vi "NOSAMSBouncerDAQ.vi"() -> (2 "Summary Data":T7 {"C12LE" format="%_3e"; "C13LE" format="%_3e"; "C1312" format="%_3e"; "C12" format="%_3e"; "C13L" format="%_3e"; "C13H" format="%_3e"}, 3 "Run Average Ratios":T8 {"LEC13/12" format="%_4e"; "DTfrac" format="%#_3g"; "DT" format="%#_3g"; "CountErr" format="%#_3g"; "d13C" format="%_4g"; "C13/12" format="%_4e"; "C14/12" format="%_4e"; "C14/13" format="%_3e"; "C12Cor" format="%_3e"; "C13" format="%_3e"; "C13H/L" format="%#_3g"})   [LabVIEW 2013]
uses:
  ctl/RunRatios.ctl
  ctl/SummaryData.ctl
  ctl/RunParameters.ctl
  ctl/PixieKeithleyDAQstates.ctl
  ctl/FCOffset.ctl
  ctl/BouncerParameters.ctl
  <vilib>/Utility/miscctls.llb/LVRowAndColumnTypeDef.ctl
  <vilib>/Utility/error.llb/DialogType.ctl
  <vilib>/DAQmx/write.llb/DAQmx Write (Analog Wfm 1Chan NSamp).vi
  <vilib>/DAQmx/read.llb/DAQmx Read (Analog 1D Wfm NChan NSamp).vi
  <vilib>/DAQmx/read.llb/DAQmx Read (Counter U32 1Chan 1Samp).vi
  <vilib>/DAQmx/create/channels.llb/DAQmx Create Channel (CI-Count Edges).vi
  <vilib>/DAQmx/create/channels.llb/DAQmx Create Channel (AI-Voltage-Basic).vi
  <vilib>/DAQmx/configure/trigger.llb/DAQmx Start Trigger (Digital Edge).vi
  <vilib>/DAQmx/configure/timing.llb/DAQmx Timing (Sample Clock).vi
  <vilib>/DAQmx/create/channels.llb/DAQmx Create Channel (AO-Voltage-Basic).vi
  <vilib>/DAQmx/configure/timing.llb/DAQmx Timing (Use Waveform).vi
  <vilib>/DAQmx/create/channels.llb/DAQmx Create Channel (CO-Pulse Generation-Time).vi
  <vilib>/DAQmx/configure/timing.llb/DAQmx Timing (Implicit).vi
  <vilib>/DAQmx/miscellaneous.llb/DAQmx Fill In Error Info.vi
  lib/PixieDriver/PixieDriver.lvlib
  <resource>/objmgr/daqmx.rc
panel:
  in  "Clear":bool
  in  "AI Samples":i32=1000
  in  "AI rate":dbl=100000.0 format="%0.2f"
  in  "Run Parameters":T1={"Block time (s)"=0.1, "Max Runtime (s)"=10.0, "Max Counts"=100000, "C12 Limit"=-1.0, "Max BadBlocks"=0, "Tuning"=FALSE, "WarmupTime"=0.0, "Warmup"=FALSE} {"Block time (s)" min=0.0 max=100.0 step=0.1}
  out "wheelfile array":string[][](array[string])=[["0", "Alfa Aesar", "N/A", "B", "30000", "180", "10", "10", "1", "", "", "", "", "", "", "", ""], ["1", "OX-I", "GS-18039", "S", "30000", "180", "10", "11", "1", "", "", "", "", "", "", "", ""], ["2", "IAEA C-1", "HY-25820", "B", "30000", "180", "10", "10", "1", "", "", "", "", "", "", "", ""], ["3", "Mullin 20150838702", "WS-32919", "U", "30000", "180", "10", "10", "1", "", "", "", "", "", "", "", ""], ["4", "Mullin 20150838703", "WS-32920", "U", "30000", "180", "10", "10", "1", "", "", "", "", "", "", "", ""], ["5", "Mullin 20150868701", "WS-32921", "U", "30000", "180", "10", "10", "1", "", "", "", "", "", "", "", ""], ["6", "Weidman Mollusc C", "HY-25773", "SS", "30000", "180", "10", "10", "1", "", "", "", "", "", "", "", ""], ["7", "OX-I", "GS-18039", "S", "30000", "180", "10", "10", "1", "", "", "", "", "", "", "", ""], ["8", "Mullin 20150928701", "WS-32922", "U", "30000", "180", "10", "10", "1", "", "", "", "", "", "", "", ""], ["9", "Mullin 20150928702", "WS-32923", "U", "30000", "180", "10", "10", "1", "", "", "", "", "", "", "", ""], ["10", "Mullin 20150928703", "WS-32924", "U", "30000", "180", "10", "10", "1", "", "", "", "", "", "", "", ""], ["11", "OX-I solid", "OC-43664", "SS", "30000", "180", "10", "10", "1", "", "", "", "", "", "", "", ""], ["12", "Mullin 20150938701", "WS-32925", "U", "30000", "180", "10", "10", "1", "", "", "", "", "", "", "", ""], ["13", "Mullin 20150938702", "WS-32926", "U", "30000", "180", "10", "10", "1", "", "", "", "", "", "", "", ""], ["14", "OX-I", "GS-18039", "S", "30000", "180", "10", "10", "1", "", "", "", "", "", "", "", ""], ["15", "Mullin 20150938703", "WS-32927", "U", "30000", "180", "10", "10", "1", "", "", "", "", "", "", "", ""], ["16", "Mullin 20150938704", "WS-32928", "U", "30000", "180", "10", "10", "1", "", "", "", "", "", "", "", ""], ["17", "Jenkins 40403", "GS-18101", "U", "30000", "180", "10", "10", "1", "", "", "", "", "", "", "", ""], ["18", "TIRI K carbonate", "HY-25794", "SS", "30000", "180", "10", "10", "1", "", "", "", "", "", "", "", ""], ["19", "Jenkins 40402", "GS-18102", "U", "30000", "180", "10", "10", "1", "", "", "", "", "", "", "", ""], ["20", "Jenkins 50412", "GS-18103", "U", "30000", "180", "10", "10", "1", "", "", "", "", "", "", "", ""], ["21", "OX-I", "GS-18039", "S", "30000", "180", "10", "10", "1", "", "", "", "", "", "", "", ""], ["22", "Jenkins 50212", "GS-18104", "U", "30000", "180", "10", "10", "1", "", "", "", "", "", "", "", ""], ["23", "Jenkins 50211", "GS-18105", "U", "30000", "180", "10", "10", "1", "", "", "", "", "", "", "", ""], ["24", "Jenkins 50210", "GS-18106", "U", "30000", "180", "10", "10", "1", "", "", "", "", "", "", "", ""], ["25", "Jenkins 50209", "GS-18108", "U", "30000", "180", "10", "10", "1", "", "", "", "", "", "", "", ""], ["26", "Jenkins 50208", "GS-18109", "U", "30000", "180", "10", "10", "1", "", "", "", "", "", "", "", ""], ["27", "OX-I", "GS-18130", "S", "30000", "180", "10", "10", "1", "", "", "", "", "", "", "", ""], ["28", "Jenkins 50207", "GS-18110", "U", "30000", "180", "10", "10", "1", "", "", "", "", "", "", "", ""], ["29", "Jenkins 50206", "GS-18111", "U", "30000", "180", "10", "10", "1", "", "", "", "", "", "", "", ""], ["30", "Jenkins 50205", "GS-18112", "U", "30000", "180", "10", "10", "1", "", "", "", "", "", "", "", ""], ["31", "TIRI I travertine", "HY-25808", "SS", "30000", "180", "10", "10", "1", "", "", "", "", "", "", "", ""], ["32", "Jenkins 50204", "GS-18120", "U", "30000", "180", "10", "10", "1", "", "", "", "", "", "", "", ""], ["33", "OX-I", "GS-17825", "S", "30000", "180", "10", "10", "1", "", "", "", "", "", "", "", ""], ["34", "Jenkins 50203", "GS-18121", "U", "30000", "180", "10", "10", "1", "", "", "", "", "", "", "", ""], ["35", "Jenkins 50202", "GS-18122", "U", "30000", "180", "10", "10", "1", "", "", "", "", "", "", "", ""], ["36", "Jenkins 50612", "GS-18123", "U", "30000", "180", "10", "10", "1", "", "", "", "", "", "", "", ""], ["37", "TIRI K carbonate", "HY-25634", "SS", "30000", "180", "10", "10", "1", "", "", "", "", "", "", "", ""], ["38", "Jenkins 50201", "GS-18124", "U", "30000", "180", "10", "10", "1", "", "", "", "", "", "", "", ""], ["39", "IAEA C-1", "HY-25820", "B", "30000", "180", "10", "10", "1", "", "", "", "", "", "", "", ""]]
  in  "Autoscale":bool=TRUE
  out "Warmup":bool
  out "C13":dbl format="%_3g"
  out "Meas":i32[](array[numeric])
  out "Runlist":i32[][](array[numeric])=[[10, 11, 10, 10, 10, 10, 10, 10, 10, 10, 10, 10, 10, 10, 10, 10, 10, 10, 10, 10, 10, 10, 10, 10, 10, 10, 10, 10, 10, 10, 10, 10, 10, 10, 10, 10, 10, 10, 10, 10]]
  in  "Clear Charts":bool
  out "LE Currents":cluster{"C13LE":dbl, "C12LE":dbl}(graph)={"C13LE"=-117.27091239941238, "C12LE"=-99.48155029506408}
  out "Currents & Counts":cluster{"C14Rate":dbl, "C12":dbl, dbl}(graph)={"C14Rate"=308.7222261479474, "C12"=134.96605939238734, 127.32704646662468}
  out "Ratios":T2(graph)={"C14/12"=1.082744261664239e-12, "C14/12"=1.1652819041526944e-12, "d13C"=-56.910193732367055, "d13C"=-56.70877952735165}
  in  "C12LE 2":dbl=1000000.0
  in  "C13LE 2":dbl=100000000.0
  in  "C13 2":dbl=100000000.0
  in  "C12 2":dbl=1000000.0
  out "Pos":i32
  in  "RowAndCollumn":T3
  in  "Numeric":i32
  in  "Start Run":bool
  in  "Tab Control":T4(tab)=enum."Status"
  in  "Load wheel":bool
  in  "Run Order":i32[](listbox)
  in  "Source Auto-shutdown":bool=TRUE
  in  "Local Results Directory":path=path "C:/Users/ams254/Documents/Results"
  out "Results path":path=path "C:/Users/ams254/Documents/Results/USAMS050815R.txt"
  out "wheelname":string caption="Wheel name"
  in  "Server Results Directory":path=path "H:/USAMS/Results"
  in  "First Run\nWarmup Multiplier":dbl=1.0 format="%#_13g"
  out "Bouncer I":waveform(dbl)(graph)={"t0"=timestamp(3552044335.624893 s since 1904-01-01), "dt"=9.999999999999972e-06, "Y"=[], "attributes"=variant("NI_ChannelName"=variant(string "PXI1Slot4/ai4"), "NI_UnitDescription"=variant(string "Volts"))}
  in  "Settings File":path
  in  "LoadSettings":bool
  in  "SaveSettings":bool
  out "HE 12C Cup":waveform(dbl)(graph)={"t0"=timestamp(3552044335.624885 s since 1904-01-01), "dt"=9.999999999999972e-06, "Y"=[], "attributes"=variant("NI_ChannelName"=variant(string "PXI1Slot4/ai0"), "NI_UnitDescription"=variant(string "Volts"))}
  out "LE 12C Cup":waveform(dbl)(graph)={"t0"=timestamp(3552044335.6252913 s since 1904-01-01), "dt"=9.999999999999972e-06, "Y"=[], "attributes"=variant("NI_ChannelName"=variant(string "PXI1Slot4/ai3"), "NI_UnitDescription"=variant(string "Volts"))}
  out "LE 13C Cup":waveform(dbl)(graph)={"t0"=timestamp(3552044335.625891 s since 1904-01-01), "dt"=9.999999999999972e-06, "Y"=[], "attributes"=variant("NI_ChannelName"=variant(string "PXI1Slot4/ai3"), "NI_UnitDescription"=variant(string "Volts"))}
  out "Bouncer V":waveform(dbl)(graph)={"t0"=timestamp(3552044335.624893 s since 1904-01-01), "dt"=9.999999999999972e-06, "Y"=[], "attributes"=variant("NI_ChannelName"=variant(string "PXI1Slot4/ai4"), "NI_UnitDescription"=variant(string "Volts"))}
  in  "FC Offset":T5={"HE 12C Offset"=-1.3999999999999993e-07, "HE 13CL Offset"=-1.6999999999999996e-10, "HE 13CH Offset"=-1.0000000000000004e-10, "LE FC Scale"=11, "HE C12 Scale"=11, "HE C13 Scale"=18} {"HE C13 Scale" items=["500 mA/V", "200 mA/V", "100 mA/V", "50 mA/V", "20 mA/V", "10 mA/V", "5 mA/V", "2 mA/V", "1 mA/V", "500 uA/V", "200 uA/V", "100 uA/V", "50 uA/V", "20 uA/V", "10 uA/V", "5 uA/V", "2 uA/V", "1 uA/V", "500 nA/V", "200 nA/V", "100 nA/V", "50 nA/V", "20 nA/V", "10 nA/V", "5 nA/V", "2 nA/V", "1 nA/V", "500 pA/V", "200 pA/V", "100 pA/V", "50 pA/V", "20 pA/V", "10 pA/V", "5 pA/V", "2 pA/V", "1 pA/V", ""]; "HE C12 Scale" items=["500 mA/V", "200 mA/V", "100 mA/V", "50 mA/V", "20 mA/V", "10 mA/V", "5 mA/V", "2 mA/V", "1 mA/V", "500 uA/V", "200 uA/V", "100 uA/V", "50 uA/V", "20 uA/V", "10 uA/V", "5 uA/V", "2 uA/V", "1 uA/V", "500 nA/V", "200 nA/V", "100 nA/V", "50 nA/V", "20 nA/V", "10 nA/V", "5 nA/V", "2 nA/V", "1 nA/V", "500 pA/V", "200 pA/V", "100 pA/V", "50 pA/V", "20 pA/V", "10 pA/V", "5 pA/V", "2 pA/V", "1 pA/V", ""]; "LE FC Scale" items=["500 mA/V", "200 mA/V", "100 mA/V", "50 mA/V", "20 mA/V", "10 mA/V", "5 mA/V", "2 mA/V", "1 mA/V", "500 uA/V", "200 uA/V", "100 uA/V", "50 uA/V", "20 uA/V", "10 uA/V", "5 uA/V", "2 uA/V", "1 uA/V", "500 nA/V", "200 nA/V", "100 nA/V", "50 nA/V", "20 nA/V", "10 nA/V", "5 nA/V", "2 nA/V", "1 nA/V", "500 pA/V", "200 pA/V", "100 pA/V", "50 pA/V", "20 pA/V", "10 pA/V", "5 pA/V", "2 pA/V", "1 pA/V", ""]; "HE 13CH Offset" format="%.1e"; "HE 13CL Offset" format="%_2e"; "HE 12C Offset" format="%_2e"}
  out "HE 13 SUM":waveform(dbl)(graph)={"t0"=timestamp(3552044335.625587 s since 1904-01-01), "dt"=9.999999999999972e-06, "Y"=[], "attributes"=variant("NI_ChannelName"=variant(string "PXI1Slot4/ai1"), "NI_UnitDescription"=variant(string "Volts"))}
  out "HE 13 Ratio":waveform(dbl)(graph)={"t0"=timestamp(3552044335.625587 s since 1904-01-01), "dt"=9.999999999999972e-06, "Y"=[], "attributes"=variant("NI_ChannelName"=variant(string "PXI1Slot4/ai1"), "NI_UnitDescription"=variant(string "Volts"))}
  in  "Bouncer Parameters":T6={"12C Period"=0.4, "12C Delay"=300.0, "12C Voltage"=11.849999999999994, "13C Period"=0.30000000000000004, "13C Delay"=200.0, "13C Voltage"=5.99999999999999, "14C Period"=100.0, "14C Delay"=800.0, "14C Voltage"=1.06, "LE13C Period"=0.19999999999999998, "LE13C Delay"=150.0, "LE13C Voltage"=1.3600000000000003, "LE12C Period"=0.20000000000000004, "LE12C Delay"=150.0, "LE12C Voltage"=6.659999999999998} {"LE12C Voltage" format="%_4f"; "LE13C Voltage" format="%_4f"; "14C Voltage" format="%_4f"; "13C Voltage" format="%_4f"; "12C Voltage" format="%_4f"}
  out "HE 13CH Cup":waveform(dbl)(graph)={"t0"=timestamp(3552044335.625587 s since 1904-01-01), "dt"=9.999999999999972e-06, "Y"=[], "attributes"=variant("NI_ChannelName"=variant(string "PXI1Slot4/ai1"), "NI_UnitDescription"=variant(string "Volts"))}
  out "HE 13CL Cup":waveform(dbl)(graph)={"t0"=timestamp(3552044335.6255894 s since 1904-01-01), "dt"=9.999999999999972e-06, "Y"=[], "attributes"=variant("NI_ChannelName"=variant(string "PXI1Slot4/ai2"), "NI_UnitDescription"=variant(string "Volts"))}
  in  "C13HLPoints":i32=10
  in  "low limit":dbl=1e-08
  out "Split Cup Good":bool=TRUE
  out "Ch0 Rate":dbl
  out "Ch0 Counts":u32
  out "Ch0 LT":dbl
  out "Ch1 Rate":dbl
  out "Ch1 Counts":u32
  out "Ch1 LT":dbl
  out "Run time [s]":dbl format="%_6g"
  out "Elapsed time":dbl format="%#_6f"
  out "Block Spectrum":u32[][](graph) caption="ADC Spectrum"
  out "CH0 SFDT":dbl format="%#_2f"
  out "CH1 SFDT":dbl format="%#_2f"
  out "SCA Counts":u32
  out "SCA Rate":dbl
  out "DT Corrected Rate Ch1":dbl
  out "CH0 GDT":dbl
  out "CH1 GDT":dbl
  out "DT Corrected Rate Ch0":dbl
  in  "CurPoints":i32=5 min=1
  in  "CountPoints":i32=5 min=1
  out "RunningAverages":T7 {"C12LE" format="%_3e"; "C13LE" format="%_3e"; "C1312" format="%_3e"; "C12" format="%_3e"; "C13L" format="%_3e"; "C13H" format="%_3e"}
  out "Moving Average Ratios":T8 {"LEC13/12" format="%_4e"; "DTfrac" format="%#_3g"; "DT" format="%#_3g"; "CountErr" format="%#_3g"; "d13C" format="%_4g"; "C13/12" format="%_4e"; "C14/12" format="%_4e"; "C14/13" format="%_3e"; "C12Cor" format="%_3e"; "C13" format="%_3e"; "C13H/L" format="%#_3g"}
  out "element":T9=enum."Stop"
  out "LoopTime":u32
  out "GetBlocktime":u32
  out "Dead time fraction":dbl
  out "Results":string[][](table)
  out "Transmission":dbl format="%#_3g"
  out "C13LE":dbl format="%_3g"
  out "C12LE":dbl format="%_3g"
  in  "Stop":bool
  in  "Stop DAQ":bool
  in  "StartDAQ":bool
  out "Good Block":bool
  out "13C H/L":dbl(knob)=0.5581291173526427 scale=0.0..2.0 scale format="%#_3g"
  out "Currents (uA)":cluster{dbl, dbl}(knob)={127.32704646662468, 134.96605939238734} scale=0.0..200.0 scale format="%#_3f"
  out "C12":dbl format="%_3g"
  out "C13L":dbl=8.662058740144909e-07 format="%_4g"
  out "C13H":dbl=4.834547199093823e-07 format="%_4g"
  # "Currents (A)"
  # "13C x100"
  # "ms"
  # "us"
  # "kV"
  # "ms"
  # "us"
  # "kV"
  # "ms"
  # "us"
  # "kV"
  # "ms"
  # "us"
  # "kV"
  # "ms"
  # "us"
  # "kV"
  # "Counts"
  # "Livetime"
  # "Rate"
  # "SFDT"
  # "GDT"
  # "Cor Rate"
  # "Ch 0"
  # "Ch1"
  # "SCA"
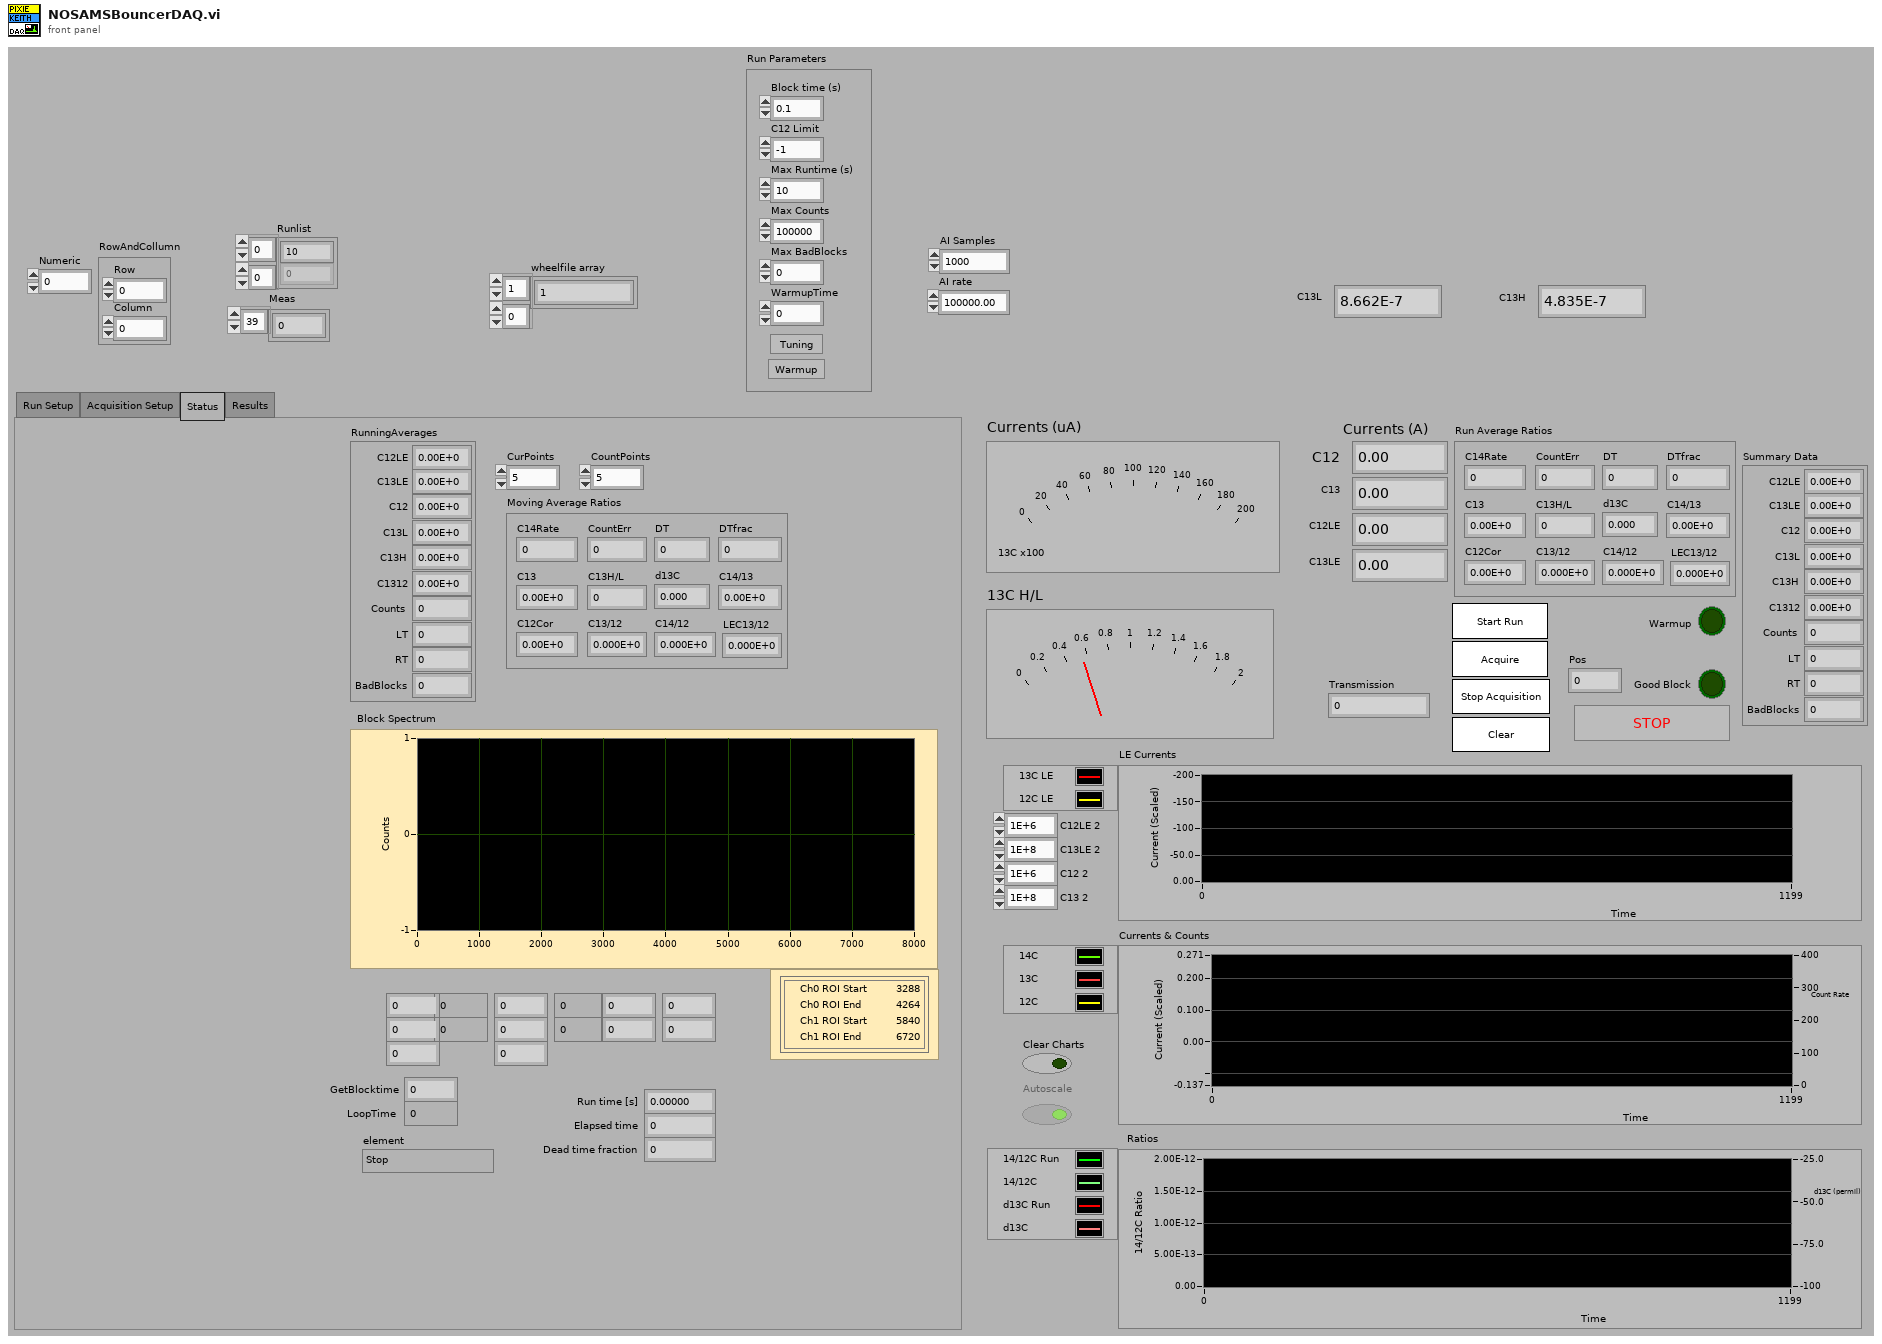
[diagram p1: front panel]
types:
  T1 = typedef "RunParameters.ctl" = cluster{"Block time (s)":dbl, "Max Runtime (s)":dbl, "Max Counts":u32, "C12 Limit":dbl, "Max BadBlocks":u8, "Tuning":bool, "WarmupTime":dbl, "Warmup":bool}
  T2 = cluster{"C14/12":dbl, "C14/12":dbl, "d13C":dbl, "d13C":dbl}
  T3 = typedef "LVRowAndColumnTypeDef.ctl" = cluster{"Row":i32, "Column":i32}
  T4 = enum32{"Run Setup", "Acquisition Setup", "Status", "Results"}
  T5 = typedef "FCOffset.ctl" = cluster{"HE 12C Offset":dbl, "HE 13CL Offset":dbl, "HE 13CH Offset":dbl, "LE FC Scale":u16, "HE C12 Scale":u16, "HE C13 Scale":u16}
  T6 = typedef "BouncerParameters.ctl" = cluster{"12C Period":dbl, "12C Delay":dbl, "12C Voltage":dbl, "13C Period":dbl, "13C Delay":dbl, "13C Voltage":dbl, "14C Period":dbl, "14C Delay":dbl, "14C Voltage":dbl, "LE13C Period":dbl, "LE13C Delay":dbl, "LE13C Voltage":dbl, "LE12C Period":dbl, "LE12C Delay":dbl, "LE12C Voltage":dbl}
  T7 = typedef "SummaryData.ctl" = cluster{"C12LE":dbl, "C13LE":dbl, "C12":dbl, "C13L":dbl, "C13H":dbl, "C1312":dbl, "Counts":u32, "LT":dbl, "RT":dbl, "BadBlocks":u8}
  T8 = typedef "RunRatios.ctl" = cluster{"C14Rate":dbl, "CountErr":dbl, "DT":dbl, "DTfrac":dbl, "C13":dbl, "C13H/L":dbl, "d13C":dbl, "C14/13":dbl, "C12Cor":dbl, "C13/12":dbl, "C14/12":dbl, "LEC13/12":dbl}
  T9 = typedef "PixieKeithleyDAQstates.ctl" = enum16{"Idle", "Initialize", "Bouncer", "Load Wheel", "Load Sample", "Start Run", "Clear", "Wait", "Get Block", "Check Data", "Check Run", "Check Sample", "Analyse and Display", "Stop DAQ", "Stop FC", "Log Data", "Stop"}
  T10 = typedef "BlockData.ctl" = cluster{"LE C12":dbl[], "LE C13":dbl[], "C12":dbl[], "C13L":dbl[], "C13H":dbl[], "C1312":dbl[], "Counts":u32[], "LT":dbl[], "RT":dbl[]}
  T11 = cluster{"C14/12":dbl, "C14/12":dbl, "d13C":dbl, "d13C":dbl}[]
  T12 = typedef "DialogType.ctl" = u16
  T13 = typedef "PixieTimes.ctl" = cluster{"CH0 LT":dbl, "CH1 LT":dbl, "CH0 SFDT":dbl, "CH1 SFDT":dbl, "CH0 GDT":dbl, "CH1 GDT":dbl, "Run time [s]":dbl}
  T14 = typedef "LVCursorListTypeDef.ctl" = cluster{"Name":string, "Color":u32, "Style":u8, "Point Style":u8, "Name Visible":bool, "Allow Drag":bool, "Cursor Mode":u32, "Plot":i32, "Index":i32, "Position":cluster{"X":dbl, "Y":dbl}, "X Scale":u32, "Y Scale":u32, "Watch Plots":i32[], "Watch All Plots":bool, "Plot Area":i32, "Label Offset":cluster{"X":dbl, "Y":dbl}}[]
  T15 = cluster{"Ch0 Counts":u32, "Ch0 Rate":dbl, "Ch0 Cor Rate":dbl, "Ch0 Cor LT":dbl, "Ch1 Counts":u32, "Ch1 Rate":dbl, "Ch1 Cor Rate":dbl, "Ch1 Cor LT":dbl}
  T16 = cluster{"index of element":i32, "element":i32, "format string":string, "format string":string}
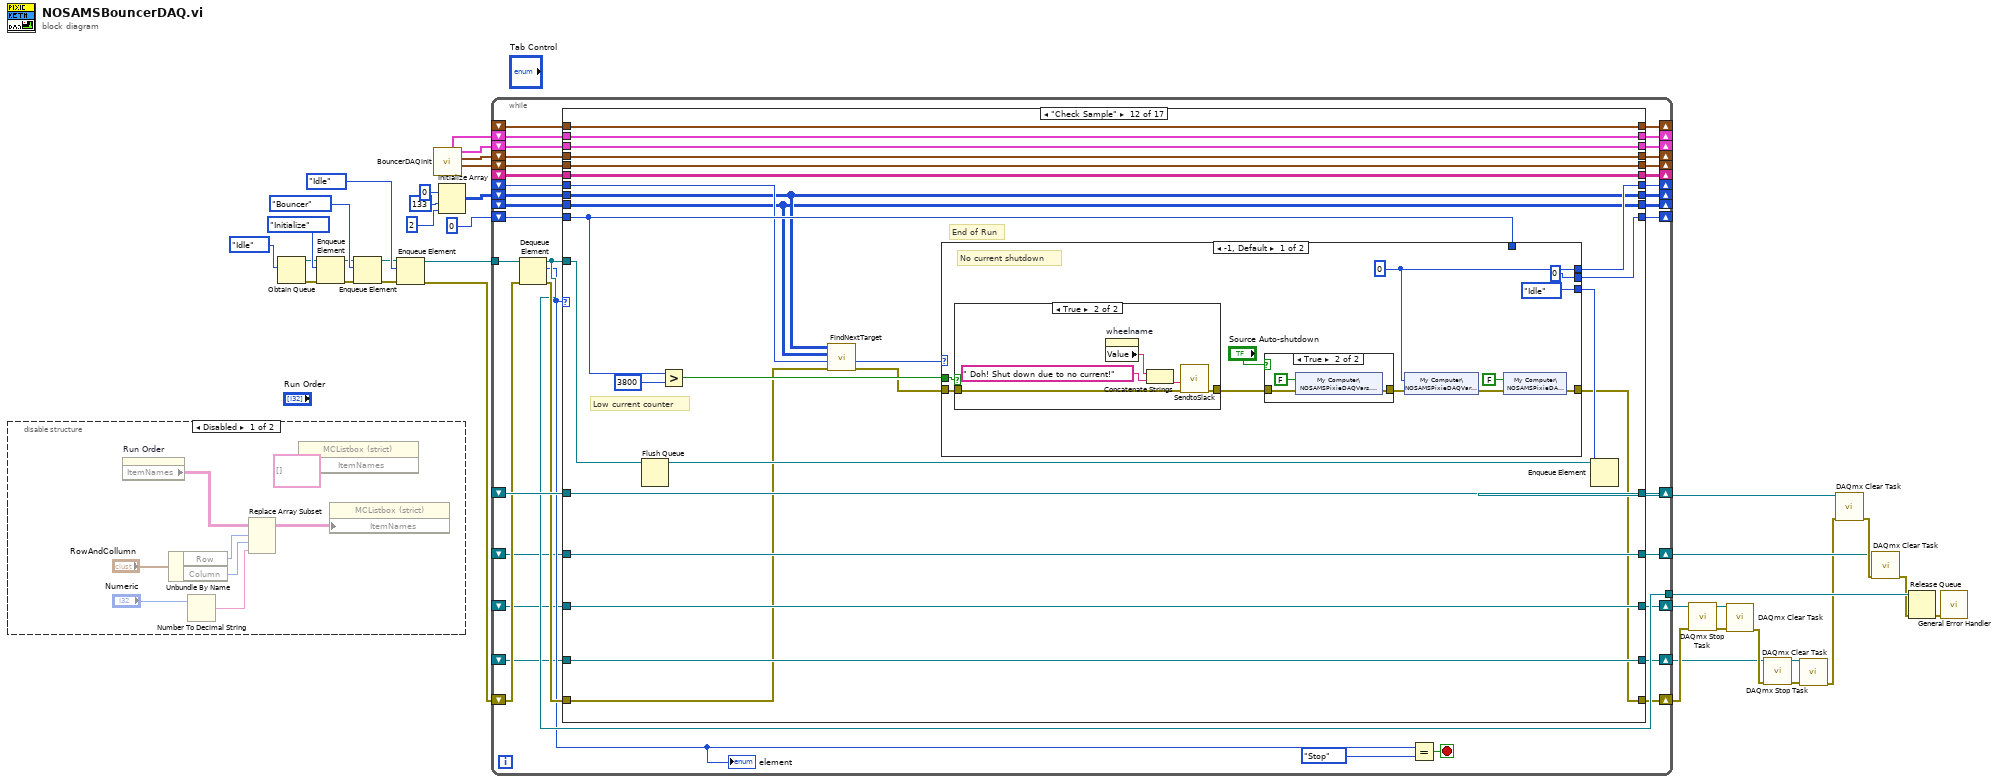
[diagram p0: block diagram]
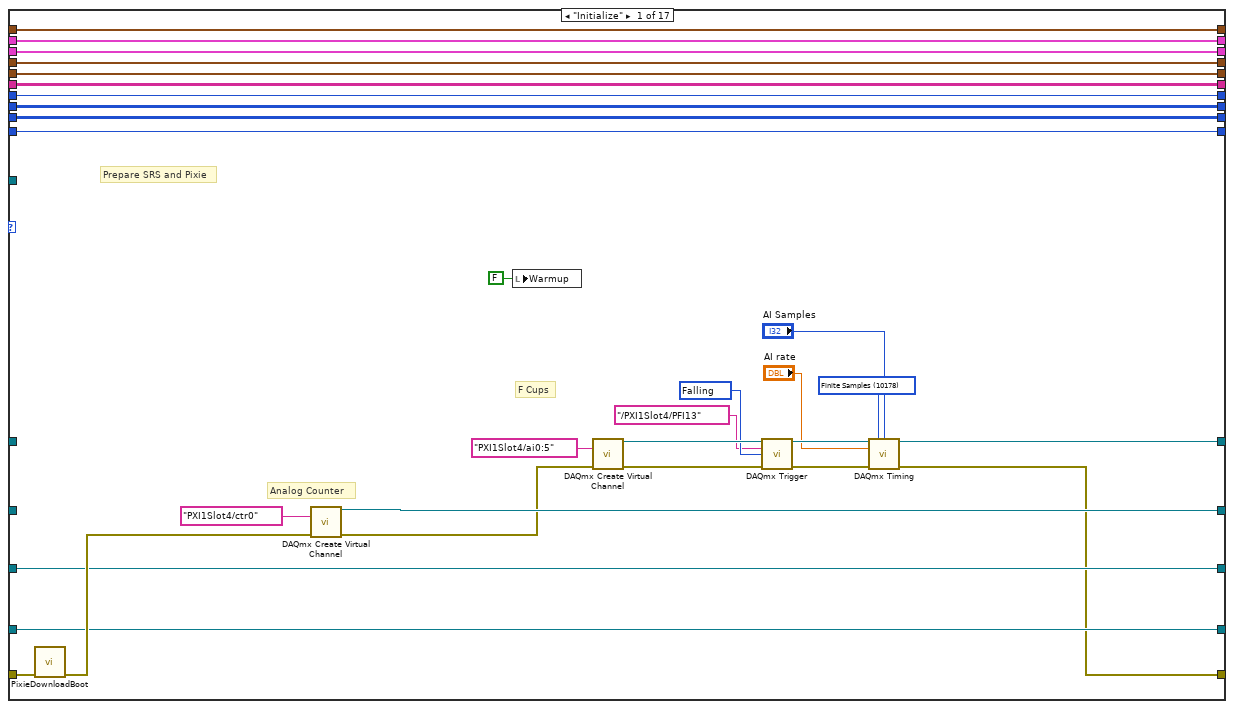
[diagram p3: hidden frame]
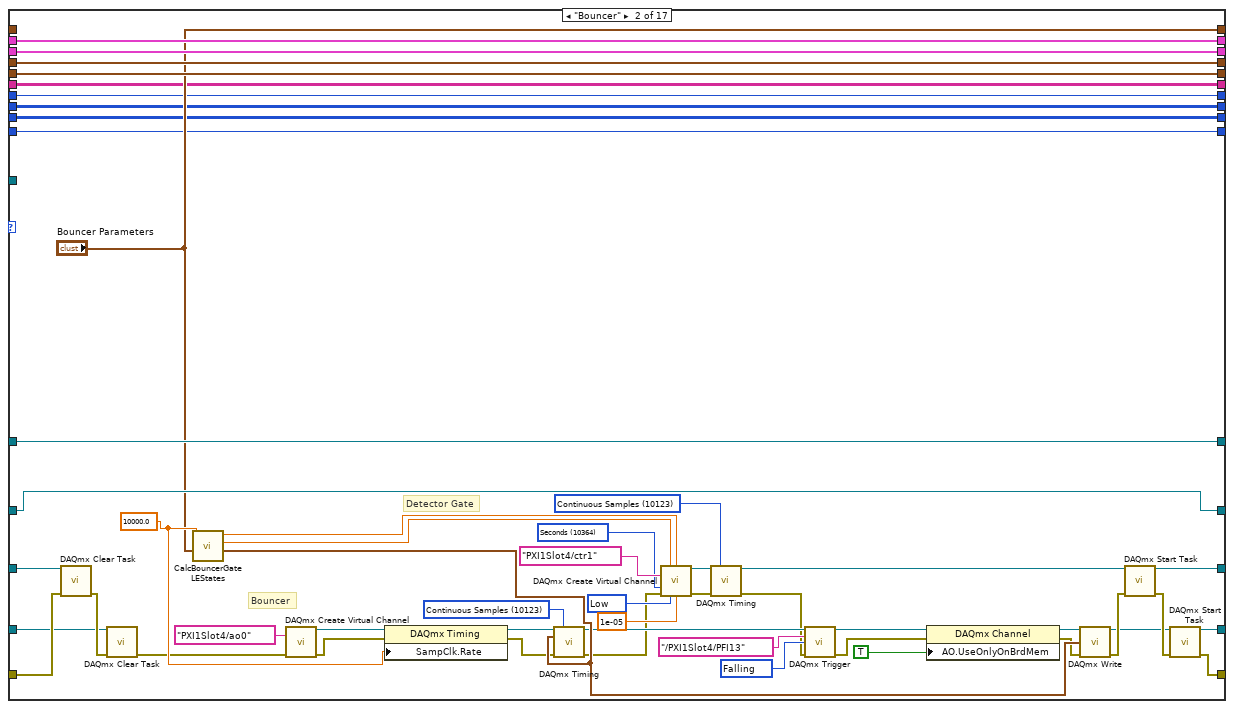
[diagram p4: hidden frame]
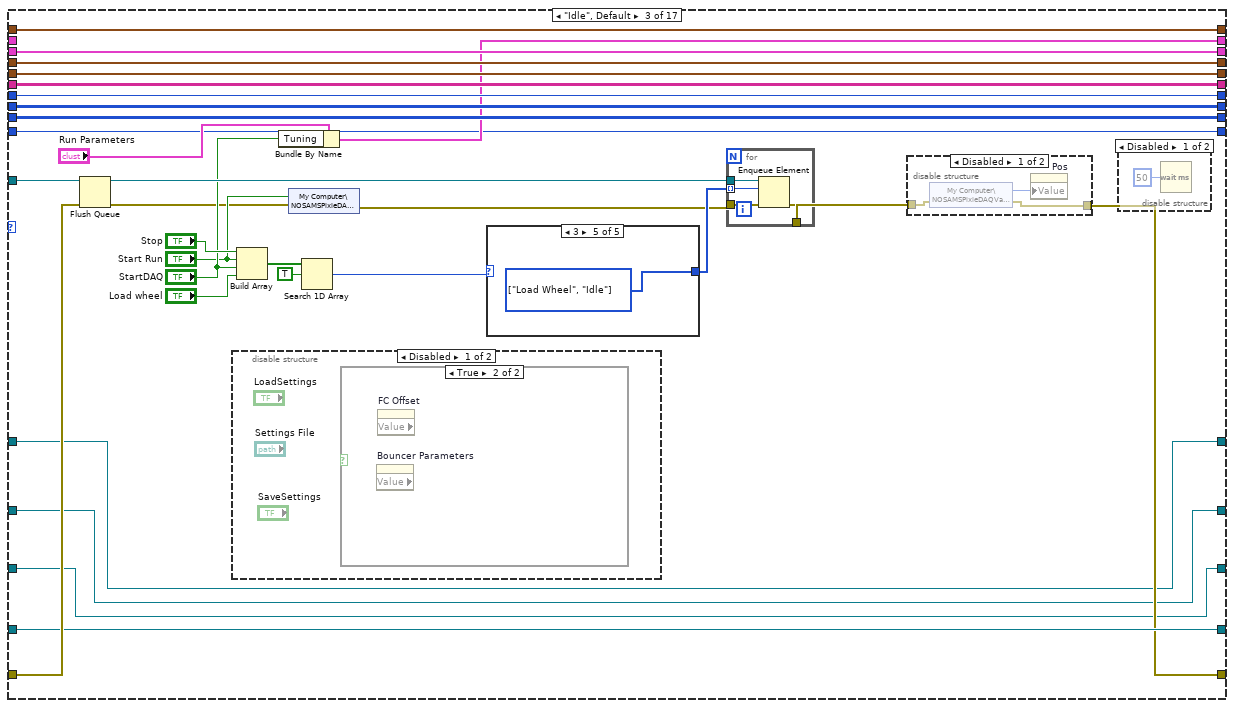
[diagram p5: hidden frame]
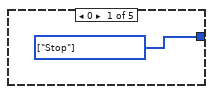
[diagram p10: hidden frame]
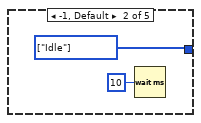
[diagram p11: hidden frame]
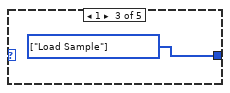
[diagram p12: hidden frame]
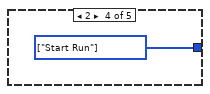
[diagram p13: hidden frame]
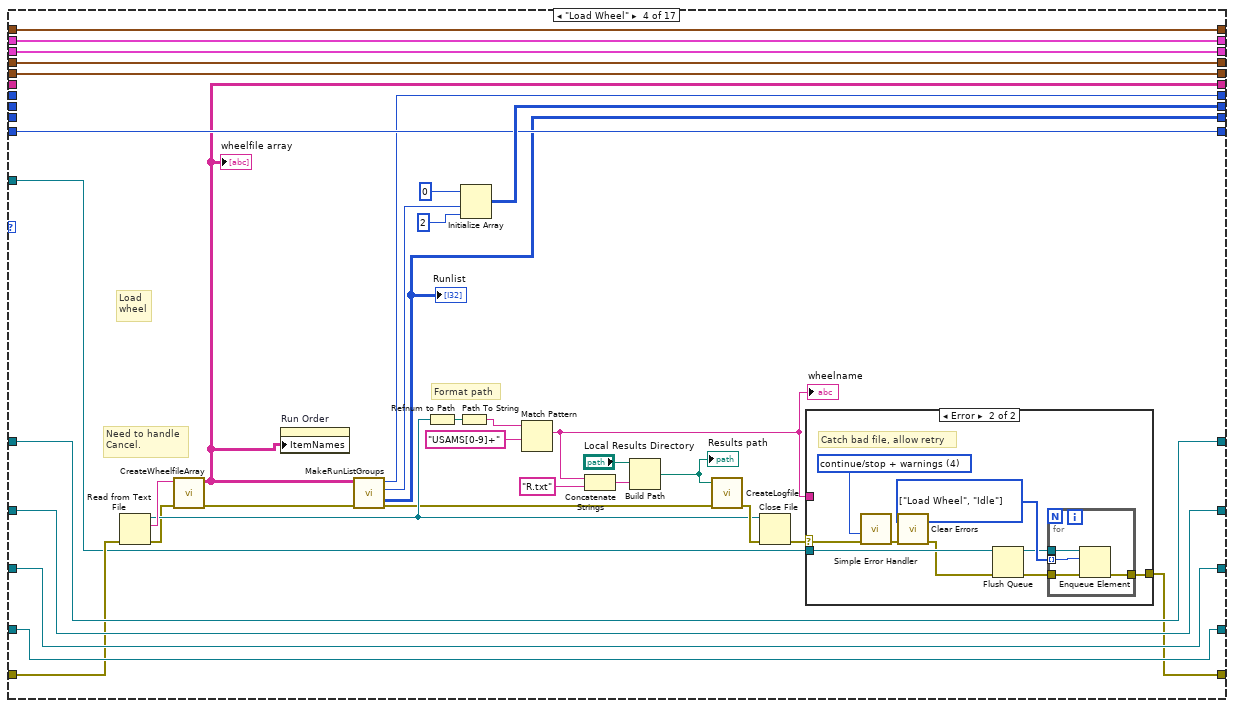
[diagram p14: hidden frame]
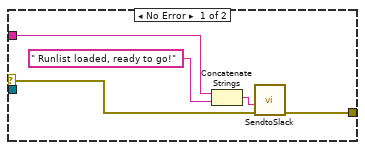
[diagram p15: hidden frame]
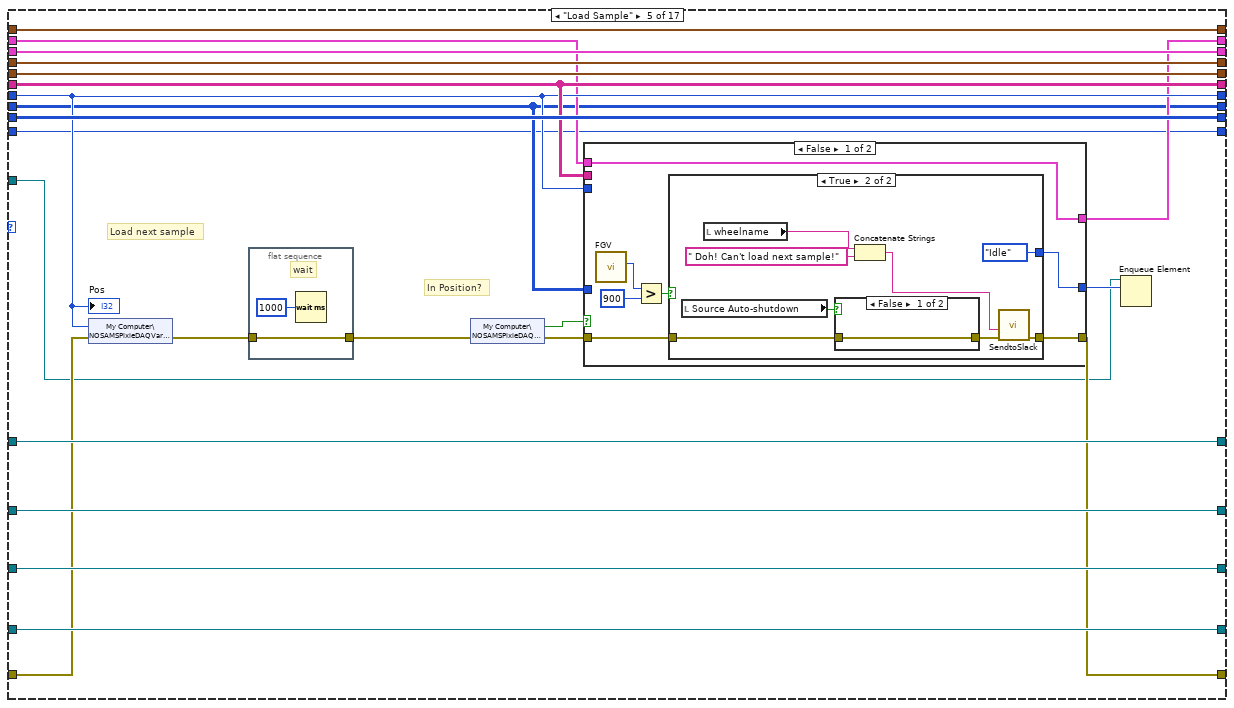
[diagram p16: hidden frame]
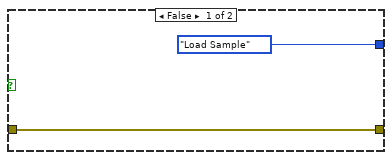
[diagram p17: hidden frame]
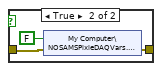
[diagram p18: hidden frame]
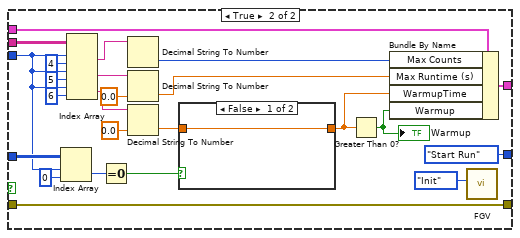
[diagram p19: hidden frame]
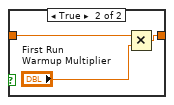
[diagram p20: hidden frame]
diagram:
  n1 = disable-structure shown="Disabled" {
    frame Disabled {
      n2 = property on="Run Order" class="MCListbox (strict)"() -> ("ItemNames"=w39:string[][])  [unwired: 2 in, 2 out]
      n3 = Unbundle By Name("RowAndCollumn") -> ("Row"=w44:i32, "Column"=w43:i32)
      n4 = Number To Decimal String(number="Numeric") -> (decimal integer string=w42:string)  [unwired: 1 out]
      n5 = Replace Array Subset(array=w39, new element=w42, index (row)=w44, index (col)=w43) -> (w38:string[][])
      n6 = property on="Property Node" class="MCListbox (strict)"("ItemNames"=string[][] [] ("Item Names")) -> ()  [unwired: 2 in, 2 out]
      n7 = property on="Property Node" class="MCListbox (strict)"("ItemNames"=w38) -> ()  [unwired: 2 in, 2 out]
    }
    frame Enabled {
    }
  }
  n8 = Obtain Queue(element data type=PixieKeithleyDAQstates."Idle" ("Next State")) -> (queue out=w29:refnum<queue>, error out=w28:errorcluster)  [unwired: 3 in, 2 out]
  n9 = Enqueue Element(queue=w29, element=PixieKeithleyDAQstates."Initialize", error in (no error)=w28) -> (queue out=w17:refnum<queue>, error out=w19:errorcluster)  [unwired: 2 out]
  n10 = Enqueue Element(queue=w17, element=PixieKeithleyDAQstates."Bouncer", error in (no error)=w19) -> (queue out=w16:refnum<queue>, error out=w18:errorcluster)  [unwired: 2 out]
  n11 = Enqueue Element(queue=w16, element=PixieKeithleyDAQstates."Idle", error in (no error)=w18) -> (queue out=w34:refnum<queue>, error out=w33:errorcluster)  [unwired: 2 out]
  n12 = call "BouncerDAQinit.vi"() -> ("Run Ratios"=w26:T8, "Summary Data"=w25:T7, "Block Data"=w24:T10, "Run Parameters"=w3:T1)  [unwired: 1 in, 7 out]
  n13 = Initialize Array(0 ("element"), 133 ("dimension size"), 2 ("dimension size")) -> (w4:i32[][])
  n14 = while {
    shift-right: [w77] -> _
    shift-left: w24 -> [w78]
    shift-right: [w75] -> _
    shift-left: w25 -> [w76]
    shift-right: [w56] -> w36
    shift-left: _ -> [w74]
    shift-right: [w47] -> w12
    shift-left: w33 -> [w71]
    tunnel: w34 -> [w73]
    tunnel: [w70] -> w31
    shift-right: [w69] -> _
    shift-left: w3 -> [w68]
    shift-right: [w65] -> _
    shift-left: w26 -> [w66]
    shift-right: [w64] -> w21
    shift-left: _ -> [w63]
    shift-right: [w62] -> w9
    shift-left: _ -> [w59]
    shift-right: [w61] -> w14
    shift-left: _ -> [w60]
    shift-right: [w58] -> _
    shift-left: _ -> [w57]
    shift-right: [w55] -> _
    shift-left: _ -> [w54]
    shift-right: [w53] -> _
    shift-left: _ -> [w51]
    shift-right: [w52] -> _
    shift-left: w4 -> [w50]
    shift-right: [w49] -> _
    shift-left: _ -> [w48]
    shift-right: [w45] -> _
    shift-left: 0 -> [w46]
    stop <- w80 stop-if-true
    n15 = Dequeue Element(queue=w73, error in (no error)=w71) -> (queue out=w70:refnum<queue>, element=w67:T9, error out=w72:errorcluster)  [unwired: 2 out]
    "element" <- w67
    n16 = case shown="\"Check Sample\"" w67 {
      tunnel: [w83 w112 w165 w215 w261 w342 w366 w405 w468 w545 w587 w662 w714 w760 w791 w822 w840] -> w47
      tunnel: w72 -> [w106 w132 w187 w227 w270 w346 w375 w449 w476 w545 w588 w659 w740 w774 w805 w819 w840]
      tunnel: w78 -> [w110 w128 w191 w232 w280 _ w385 w436 w478 w558 w608 w677 w725 w780 w811 w836 w855]
      tunnel: [w110 w128 w191 w232 w280 w339 w385 w459 w477 w558 w608 w677 w725 w780 w811 w836 w855] -> w77
      tunnel: w76 -> [w109 w127 w190 w231 w281 _ w384 w435 w480 w556 w633 w676 w724 w779 w810 w835 w854]
      tunnel: [w109 w127 w190 w231 w281 w338 w384 w435 w479 w556 w633 w676 w724 w779 w810 w835 w854] -> w75
      tunnel: w68 -> [w105 w129 _ w233 w266 w335 w383 w455 w485 w526 w636 w678 w746 w763 w794 w837 w850]
      tunnel: w74 -> [_ w125 w162 w235 w276 w358 w377 w461 w473 w535 w614 w672 w748 w775 w806 w829 w851]
      tunnel: w70 -> [_ _ w189 w214 w260 w341 w373 _ w486 w534 _ w673 _ w776 w807 _ w852]
      tunnel: [w105 w129 w172 w233 w265 w335 w383 w455 w485 w525 w636 w678 w746 w763 w794 w837 w850] -> w69
      tunnel: w66 -> [w104 w126 w185 w230 w282 _ w382 w454 w483 w552 _ w675 w723 w773 w804 w834 w849]
      tunnel: [w104 w126 w185 w230 w282 w337 w382 w454 w483 w552 w635 w675 w723 w773 w804 w834 w849] -> w65
      tunnel: [w102 w124 w163 w236 w275 w351 w381 w425 w474 w536 w606 w671 w742 w772 w803 w824 w848] -> w64
      tunnel: w63 -> [_ w124 w163 w236 w275 w352 w381 w425 w474 w536 w606 w671 w745 w772 w803 w825 w848]
      tunnel: [w89 w118 w184 w238 w273 w348 w379 w448 w482 w551 w634 w669 w734 w770 w801 w826 w846] -> w62
      tunnel: [w90 w121 w164 w237 w274 w349 w380 w426 w475 w537 w607 w670 w735 w771 w802 w827 w847] -> w61
      tunnel: w60 -> [w90 w130 w164 w237 w274 w349 w380 w426 w475 w537 w607 w670 w735 w771 w802 w827 w847]
      tunnel: w59 -> [w89 w131 w184 w238 w273 w348 w379 w448 w482 w551 w634 w669 w734 w770 w801 w826 w846]
      tunnel: [w88 "Bouncer Parameters" w183 w234 w279 w347 w378 w444 w481 w550 w632 w679 w733 w769 w800 w838 w845] -> w58
      tunnel: w57 -> [w88 _ w183 w234 w279 w347 w378 w444 w481 w550 w632 w679 w733 w769 w800 w838 w845]
      tunnel: [w91 w125 w162 w235 w276 w357 w376 w424 w473 w535 w614 w672 w747 w775 w806 w828 w851] -> w56
      tunnel: [w87 w116 w177 w209 w268 w343 w370 w409 w472 w548 w613 w661 w727 w764 w795 w833 w844] -> w55
      tunnel: w54 -> [w87 w116 w177 _ w268 w343 w370 w409 w472 w548 w613 w661 w727 w764 w795 w833 w844]
      tunnel: [w86 w115 w176 w210 w267 w336 w369 w408 w471 w547 w612 w667 w710 w765 w796 w832 w843] -> w53
      tunnel: [w85 w114 w175 w228 w264 w345 w368 w407 w470 w540 w611 w656 w712 w766 w797 w831 w842] -> w52
      tunnel: w51 -> [w86 w115 w176 _ w267 w336 w369 w408 w471 w547 w612 w657 w710 w765 w796 w832 w843]
      tunnel: w50 -> [w85 w114 w175 _ w264 w345 w368 w407 w470 w549 w611 w656 w712 w766 w797 w831 w842]
      tunnel: [w84 w113 w174 w207 w277 w344 w367 w406 w469 w546 w610 w655 w726 w767 w798 w830 w841] -> w49
      tunnel: w48 -> [w84 w113 w174 _ w277 w344 w367 w406 w469 w546 w610 w655 w726 w767 w798 w830 w841]
      tunnel: w46 -> [w82 w111 w170 w224 w263 w334 w365 w401 w467 w541 w600 w663 w722 w762 w793 w821 w839]
      tunnel: [w82 w111 w170 w224 w263 w334 w365 w401 w467 w541 w598 w664 w722 w762 w793 w821 w839] -> w45
      frame "Initialize" {
        w96 = 10171 items=["Rising"=10280, "Falling"=10171] ("edge")
        w107 = 10178 items=["Finite Samples"=10178, "Continuous Samples"=10123] ("sample mode")
        # "Analog Counter"
        # "F Cups"
        # "Prepare SRS and Pixie"
        n17 = call "PixieDownloadBoot.vi"("error in (no error)"=w106) -> ("error out"=w94:errorcluster)  [unwired: 5 in, 5 out]
        n18 = call-poly <vilib>:"DAQmx Create Virtual Channel.vi"("counter"=tag "PXI1Slot4/ctr0" ("Counter(s)"), "error in"=w94) -> ("task out"=w102:refnum<k21>, "error out"=w101:errorcluster)  [unwired: 5 in, 7 out]
        n19 = local write "Warmup"(FALSE ("Warmup")) -> ()
        n20 = call-poly <vilib>:"DAQmx Create Virtual Channel.vi"("physical channels"=tag "PXI1Slot4/ai0:5", "error in"=w101) -> ("task out"=w100:refnum<k21>, "error out"=w98:errorcluster)  [unwired: 7 in, 5 out]
        n21 = call-poly <vilib>:"DAQmx Trigger.vi"("task/channels in"=w100, "source"=tag "/PXI1Slot4/PFI13", "edge"=w96, "error in"=w98) -> ("task out"=w99:refnum<k21>, "error out"=w97:errorcluster)  [unwired: 10 in]
        n22 = call-poly <vilib>:"DAQmx Timing.vi"("task/channels in"=w99, "sample mode"=w107, "samples per channel"="AI Samples", "rate"="AI rate", "error in"=w97) -> ("task out"=w91:refnum<k21>, "error out"=w83:errorcluster)  [unwired: 2 in, 7 out]
      }
      frame "Bouncer" {
        w148 = 10171 items=["Rising"=10280, "Falling"=10171] ("edge")
        w146 = 10123 items=["Finite Samples"=10178, "Continuous Samples"=10123] ("sample mode")
        w143 = 10123 items=["Finite Samples"=10178, "Continuous Samples"=10123, "Hardware Timed Single Point"=12522] ("sample mode")
        w138 = 10214 items=["High"=10192, "Low"=10214] ("idle state")
        w139 = 10364 items=["Seconds"=10364] ("units")
        w161 = 10000.0 ("rate")
        # "Bouncer"
        # "Detector Gate"
        n23 = call <vilib>:"DAQmx Clear Task.vi"("task in"=w130, "error in"=w132) -> ("error out"=w133:errorcluster)  [unwired: 13 in]
        n24 = call <vilib>:"DAQmx Clear Task.vi"("task in"=w131, "error in"=w133) -> ("error out"=w134:errorcluster)  [unwired: 13 in]
        n25 = call "CalcBouncerGateLEStates.vi"("Bouncer Settings"="Bouncer Parameters", "SampClk.Rate"=w161) -> ("Bouncer Waveform"=w160:waveform(dbl), "High time"=w145:dbl, "low time"=w144:dbl)  [unwired: 7 in]
        n26 = call-poly <vilib>:"DAQmx Create Virtual Channel.vi"("physical channels"=tag "PXI1Slot4/ao0", "error in"=w134) -> ("task out"=w156:refnum<k21>, "error out"=w155:errorcluster)  [unwired: 7 in, 5 out]
        n27 = property class="DAQmx Timing"(reference=w156, error in=w155, "SampClk.Rate"=w161) -> (reference out=w157:refnum<k21>, error out=w158:errorcluster)
        n28 = call-poly <vilib>:"DAQmx Timing.vi"("task/channels in"=w157, "sample mode"=w146, "waveform"=w160, "error in"=w158) -> ("task out"=w147:refnum<k21>, "error out"=w136:errorcluster)  [unwired: 10 out]
        n29 = call-poly <vilib>:"DAQmx Create Virtual Channel.vi"("high time"=w145, "low time"=w144, "counter"=tag "PXI1Slot4/ctr1", "units"=w139, "error in"=w136, "idle state"=w138, "initial delay"=1e-05) -> ("task out"=w142:refnum<k21>, "error out"=w141:errorcluster)  [unwired: 2 in, 5 out]
        n30 = call-poly <vilib>:"DAQmx Timing.vi"("task/channels in"=w142, "sample mode"=w143, "error in"=w141) -> ("task out"=w122:refnum<k21>, "error out"=w135:errorcluster)  [unwired: 1 in, 10 out]
        n31 = call-poly <vilib>:"DAQmx Trigger.vi"("task/channels in"=w147, "source"=tag "/PXI1Slot4/PFI13", "edge"=w148, "error in"=w135) -> ("task out"=w151:refnum<k21>, "error out"=w153:errorcluster)  [unwired: 10 out]
        n32 = property class="DAQmx Channel"(reference=w151, error in=w153, "AO.UseOnlyOnBrdMem"=TRUE) -> (reference out=w152:refnum<k21>, error out=w154:errorcluster)
        n33 = call-poly <vilib>:"DAQmx Write.vi"("task/channels in"=w152, "data"=w160, "error in"=w154) -> ("task out"=w119:refnum<k21>, "error out"=w120:errorcluster)  [unwired: 1 in, 10 out]
        n34 = call <vilib>:"DAQmx Start Task.vi"("task/channels in"=w122, "error in"=w120) -> ("task out"=w121:refnum<k21>, "error out"=w123:errorcluster)  [unwired: 12 in]
        n35 = call <vilib>:"DAQmx Start Task.vi"("task/channels in"=w119, "error in"=w123) -> ("task out"=w118:refnum<k21>, "error out"=w112:errorcluster)  [unwired: 12 in]
      }
      frame "Idle", Default {
        n36 = Flush Queue(queue=w189, error in (no error)=w187) -> (queue out=w186:refnum<queue>, error out=w168:errorcluster)  [unwired: 1 out]
        n37 = disable-structure shown="Disabled" {
          frame Disabled {
            n38 = case shown="True" {
              selector: _ -> [_ _]
              frame False {
              }
              frame True {
                n39 = property on="Bouncer Parameters" class="Clust (strict)" props=["Value"]() -> ()  [unwired: 2 in, 3 out]
                n40 = property on="FC Offset" class="Clust (strict)" props=["Value"]() -> ()  [unwired: 2 in, 3 out]
              }
            }
          }
          frame Enabled {
          }
        }
        n41 = Build Array("Stop", "Start Run", "StartDAQ", "Load wheel") -> (w180:bool[])
        n42 = Bundle By Name(cluster="Run Parameters", "Tuning"="StartDAQ") -> (w172:T1)
        n43 = shared-variable "My Computer\\NOSAMSPixieDAQVars.lvlib\\Auto"("Start Run", error in=w168) -> (error out=w167:errorcluster)
        n44 = Search 1D Array(1D array=w180, element=TRUE) -> (index of element=w178:i32)  [unwired: 1 in]
        n45 = case shown="3" w178 {
          tunnel: [w201 w202 w204 w205 w206] -> w188
          frame 0 {
            w201 = T9[] [enum."Stop"] items=["Idle", "Initialize", "Bouncer", "Load Wheel", "Load Sample", "Start Run", "Clear", "Wait", "Get Block", "Check Data", "Check Run", "Check Sample", "Analyse and Display", "Stop DAQ", "Stop FC", "Log Data", "Stop"]
          }
          frame -1, Default {
            w202 = T9[] [enum."Idle"] items=["Idle", "Initialize", "Bouncer", "Load Wheel", "Load Sample", "Start Run", "Clear", "Wait", "Get Block", "Check Data", "Check Run", "Check Sample", "Analyse and Display", "Stop DAQ", "Stop FC", "Log Data", "Stop"]
            n46 = Wait (ms)(milliseconds to wait=u32 10) -> ()  [unwired: 1 out]
          }
          frame 1 {
            w204 = T9[] [enum."Load Sample"] items=["Idle", "Initialize", "Bouncer", "Load Wheel", "Load Sample", "Start Run", "Clear", "Wait", "Get Block", "Check Data", "Check Run", "Check Sample", "Analyse and Display", "Stop DAQ", "Stop FC", "Log Data", "Stop"]
          }
          frame 2 {
            w205 = T9[] [enum."Start Run"] items=["Idle", "Initialize", "Bouncer", "Load Wheel", "Load Sample", "Start Run", "Clear", "Wait", "Get Block", "Check Data", "Check Run", "Check Sample", "Analyse and Display", "Stop DAQ", "Stop FC", "Log Data", "Stop"]
          }
          frame 3 {
            w206 = T9[] [enum."Load Wheel", enum."Idle"] items=["Idle", "Initialize", "Bouncer", "Load Wheel", "Load Sample", "Start Run", "Clear", "Wait", "Get Block", "Check Data", "Check Run", "Check Sample", "Analyse and Display", "Stop DAQ", "Stop FC", "Log Data", "Stop"]
          }
        }
        n47 = for {
          tunnel: w188 -> [w200] mode=indexing
          tunnel: [w199] -> w166
          tunnel: w186 -> [w198]
          tunnel: w167 -> [w197]
          n48 = Enqueue Element(queue=w198, element=w200, error in (no error)=w197) -> (error out=w199:errorcluster)  [unwired: 3 out]
        }
        n49 = disable-structure shown="Disabled" {
          disable-tunnel: w166 -> [w194 w196]
          disable-tunnel: [w193 w196] -> w165
          frame Disabled {
            n50 = shared-variable "My Computer\\NOSAMSPixieDAQVars.lvlib\\CurPos"(error in=w194) -> (w195:i32, error out=w193:errorcluster)
            n51 = property on="Pos" class="DigNum (strict)"("Value"=w195) -> ()  [unwired: 2 in, 2 out]
          }
          frame Enabled {
          }
        }
        n52 = disable-structure shown="Disabled" {
          frame Disabled {
            n53 = Wait (ms)(milliseconds to wait=u32 50) -> ()  [unwired: 1 out]
          }
          frame Enabled {
          }
        }
      }
      frame "Load Wheel" {
        # "Need to handle\nCancel."
        # "Format path"
        # "Load\nwheel"
        n54 = Read from Text File(error in=w227) -> (refnum out=w225:refnum<file>, text=w240:string, error out=w218:errorcluster)  [unwired: 4 out]
        n55 = call "CreateWheelfileArray.vi"("error in (no error)"=w218, "Wheelfile"=w240) -> ("error out"=w213:errorcluster, "Wheelfile Array"=w209:string[][])  [unwired: 8 in]
        "wheelfile array" <- w209
        n56 = property on="Run Order" class="MCListbox (strict)"("ItemNames"=w209) -> ()  [unwired: 2 in, 2 out]
        n57 = call "MakeRunListGroups.vi"("error in"=w213, "WheelList"=w209) -> ("error out"=w212:errorcluster, "Runlist"=w207:i32[][], "SampleCount"=w211:i32, "First Sample"=w210:i32)  [unwired: 5 in]
        "Runlist" <- w207
        n58 = Refnum to Path(1:w225) -> (0:w241:path)
        n59 = Path To String(path=w241) -> (string=w219:string)
        n60 = Initialize Array(0 ("element"), w211, 2 ("dimension size")) -> (w228:i32[][])
        n61 = Match Pattern(string=w219, regular expression="USAMS[0-9]+") -> (match substring=w216:string)  [unwired: 4 out]
        "wheelname" <- w216
        n62 = Concatenate Strings(w216, "R.txt") -> (w221:string)
        n63 = Build Path(base path="Local Results Directory", name or relative path=w221) -> (appended path=w220:path)
        "Results path" <- w220
        n64 = call "CreateLogfile.vi"("error in (no error)"=w212, "Log File Path"=w220) -> ("error out"=w226:errorcluster)  [unwired: 9 in]
        n65 = Close File(refnum=w225, error in=w226) -> (error out=w217:errorcluster)  [unwired: 1 out]
        n66 = case shown="Error" w217 {
          selector: w217 -> [w244 w255]
          tunnel: [w245 w251] -> w215
          tunnel: w216 -> [w243 _]
          tunnel: w214 -> [_ w249]
          frame No Error {
            n67 = Concatenate Strings(w243, " Runlist loaded, ready to go!") -> (w246:string)
            n68 = call "SendtoSlack.vi"("error in (no error)"=w244, "buffer"=w246) -> ("error out"=w245:errorcluster)  [unwired: 7 in, 2 out]
          }
          frame Error {
            w253 = T9[] [enum."Load Wheel", enum."Idle"] items=["Idle", "Initialize", "Bouncer", "Load Wheel", "Load Sample", "Start Run", "Clear", "Wait", "Get Block", "Check Data", "Check Run", "Check Sample", "Analyse and Display", "Stop DAQ", "Stop FC", "Log Data", "Stop"]
            w254 = T12 4 items=["no dialog", "OK message", "continue or stop message", "OK message + warnings", "continue/stop + warnings"] ("type of dialog (OK msg:1)")
            # "Catch bad file, allow retry"
            n69 = call <vilib>:"Simple Error Handler.vi"("type of dialog (OK msg:1)"=w254, "error in (no error)"=w255) -> ("error out"=w248:errorcluster)  [unwired: 3 in, 4 out]
            n70 = call <vilib>:"Clear Errors.vi"("error in (no error)"=w248) -> ("error out"=w247:errorcluster)  [unwired: 6 in]
            n71 = Flush Queue(queue=w249, error in (no error)=w247) -> (queue out=w250:refnum<queue>, error out=w252:errorcluster)  [unwired: 1 out]
            n72 = for {
              tunnel: [w259] -> w251
              tunnel: w253 -> [w258] mode=indexing
              tunnel: w252 -> [w257]
              tunnel: w250 -> [w256]
              n73 = Enqueue Element(queue=w256, element=w258, error in (no error)=w257) -> (error out=w259:errorcluster)  [unwired: 3 out]
            }
          }
        }
      }
      frame "Load Sample" {
        # "Load next sample"
        # "In Position?"
        n74 = shared-variable "My Computer\\NOSAMSPixieDAQVars.lvlib\\PosReq"(w267, error in=w270) -> (error out=w272:errorcluster)
        n75 = flat-sequence {
          tunnel: [w283] -> w271
          tunnel: w272 -> [w283]
          frame #0 {
            # "wait"
            n76 = Wait (ms)(milliseconds to wait=u32 1000) -> ()  [unwired: 1 out]
          }
        }
        n77 = shared-variable "My Computer\\NOSAMSPixieDAQVars.lvlib\\InPos"(error in=w271) -> (w269:bool, error out=w262:errorcluster)
        n78 = case shown="False" w269 {
          tunnel: [w291 PixieKeithleyDAQstates."Start Run" ("element")] -> w278
          tunnel: w268 -> [_ w318]
          tunnel: w267 -> [_ w314]
          tunnel: w266 -> [w288 w317]
          tunnel: [w288 w316] -> w265
          tunnel: w264 -> [_ w315]
          tunnel: [w290 w311] -> w261
          tunnel: w262 -> [w289 w311]
          frame False {
            n79 = call "FGV.vi"() -> ("Iterations"=w285:u32)  [unwired: 10 in, 1 out]
            n80 = Greater?(x=w285, y=u32 900) -> (0:w287:bool)
            n81 = case shown="True" w287 {
              tunnel: [PixieKeithleyDAQstates."Load Sample" ("element") PixieKeithleyDAQstates."Idle" ("element")] -> w291
              tunnel: [w292 w298] -> w290
              tunnel: w289 -> [w292 w296]
              frame False {
              }
              frame True {
                n82 = local read "Source Auto-shutdown"() -> (w295:bool)
                n83 = local read "wheelname"() -> (w294:string)
                n84 = case shown="False" w295 {
                  tunnel: [w302 w304] -> w297
                  tunnel: w296 -> [w302 w303]
                  frame False {
                  }
                  frame True {
                    n85 = shared-variable "My Computer\\NOSAMSPixieDAQVars.lvlib\\ResEnable"(FALSE ("ResEnable"), error in=w303) -> (error out=w304:errorcluster)
                  }
                }
                n86 = Concatenate Strings(w294, " Doh! Can't load next sample!" ("string")) -> (w299:string)
                n87 = call "SendtoSlack.vi"("error in (no error)"=w297, "buffer"=w299) -> ("error out"=w298:errorcluster)  [unwired: 7 in, 2 out]
              }
            }
          }
          frame True {
            n88 = Index Array(array=w315, index (row)=w314, index (col)=0 ("disabled index (col)")) -> (element=w313:i32)
            n89 = Index Array(array=w318, index (row) #1=w314, index (col) #1=4 ("disabled index (col)"), index (row) #2=w314, index (col) #2=5 ("disabled index (col)"), index (row) #3=w314, index (col) #3=6 ("disabled index (col)")) -> (element #1=w325:string, element #2=w326:string, element #3=w319:string)
            n90 = Equal To 0?(x=w313) -> (x = 0?=w309:bool)
            n91 = Decimal String To Number(string=w325) -> (number=w324:i32)  [unwired: 2 in, 1 out]
            n92 = Decimal String To Number(string=w326, default (0L)=0.0 ("default (0 I32)")) -> (number=w323:dbl)  [unwired: 1 in, 1 out]
            n93 = Decimal String To Number(string=w319, default (0L)=0.0 ("default (0 I32)")) -> (number=w308:dbl)  [unwired: 1 in, 1 out]
            n94 = case shown="False" w309 {
              tunnel: w308 -> [w330 w333]
              tunnel: [w330 w331] -> w307
              frame False {
              }
              frame True {
                n95 = Multiply(x=w333, y="First Run\nWarmup Multiplier") -> (x*y=w331:dbl)
              }
            }
            n96 = Greater Than 0?(x=w307) -> (x > 0?=w306:bool)
            "Warmup" <- w306
            n97 = Bundle By Name(cluster=w317, "Max Counts"=w324, "Max Runtime (s)"=w323, "WarmupTime"=w307, "Warmup"=w306) -> (w316:T1)
            n98 = call "FGV.vi"("Mode (Update)"=enum16{"Update", "Init"}."Init") -> ()  [unwired: 9 in, 2 out]
          }
        }
        n99 = Enqueue Element(queue=w260, element=w278) -> ()  [unwired: 2 in, 3 out]
        "Pos" <- w267
      }
      frame "Start Run" {
        w353 = T9[] [enum."Wait", enum."Get Block", enum."Check Data"] items=["Idle", "Initialize", "Bouncer", "Load Wheel", "Load Sample", "Start Run", "Clear", "Wait", "Get Block", "Check Data", "Check Run", "Check Sample", "Analyse and Display", "Stop DAQ", "Stop FC", "Log Data", "Stop"]
        # "Start Bouncer and Gate\nTrigger DAQ and PIXIE"
        # "Start counter"
        # "Code to trigger sync start goes here"
        # "Start/trigger PIXIE"
        # "Start FC DAQ"
        n100 = Flush Queue(queue=w341) -> (queue out=w340:refnum<queue>)  [unwired: 1 in, 2 out]
        n101 = call "BouncerDAQinit.vi"() -> ("Run Ratios"=w337:T8, "Summary Data"=w338:T7, "Block Data"=w339:T10)  [unwired: 1 in, 8 out]
        n102 = call <vilib>:"DAQmx Start Task.vi"("task/channels in"=w358, "error in"=w346) -> ("task out"=w357:refnum<k21>, "error out"=w360:errorcluster)  [unwired: 12 out]
        n103 = call "PixieStartACQ.vi"("error in (no error)"=w346) -> ("error out"=w359:errorcluster)  [unwired: 2 in, 8 out]
        n104 = call <vilib>:"DAQmx Start Task.vi"("task/channels in"=w352, "error in"=w346) -> ("task out"=w351:refnum<k21>, "error out"=w350:errorcluster)  [unwired: 12 out]
        n105 = call "ElapsedTime.vi"("error in (no error)"=w346, "Mode (Update)"=enum16{"Update", "Init"}."Init") -> ("error out"=w356:errorcluster)  [unwired: 9 out]
        n106 = Merge Errors(w356, w359, w360, w350) -> (w354:errorcluster)
        n107 = for {
          tunnel: w340 -> [w364]
          tunnel: w354 -> [w363]
          tunnel: [w362] -> w342
          tunnel: w353 -> [w361] mode=indexing
          n108 = Enqueue Element(queue=w364, element=w361, error in (no error)=w363) -> (error out=w362:errorcluster)  [unwired: 3 out]
        }
      }
      frame "Wait" {
        # "Handle errors here?"
        n109 = event shown="[1] \"Bouncer Parameters\": Value Change" {
          selector: _ -> [_ _]
          dyn-events: _ -> [_ _]
          timeout: 0 -> [_ _]
          tunnel: w377 -> [w389 w391]
          tunnel: [w388 w391] -> w376
          tunnel: w375 -> [w387 w393]
          tunnel: [w386 w392] -> w371
          tunnel: w373 -> [_ w390]
          event Timeout {
            n110 = event-data() -> ()  [unwired: 1 in, 2 out]
            n111 = call <vilib>:"DAQmx Wait Until Done.vi"("task/channels in"=w389, "error in"=w387) -> ("task out"=w388:refnum<k21>, "error out"=w386:errorcluster)  [unwired: 12 in]
          }
          event Value Change {
            w394 = T9[] [enum."Bouncer", enum."Wait"] items=["Idle", "Initialize", "Bouncer", "Load Wheel", "Load Sample", "Start Run", "Clear", "Wait", "Get Block", "Check Data", "Check Run", "Check Sample", "Analyse and Display", "Stop DAQ", "Stop FC", "Log Data", "Stop"]
            n112 = event-data() -> ()  [unwired: 1 in, 5 out]
            n113 = for {
              tunnel: w390 -> [w398]
              tunnel: w393 -> [w397]
              tunnel: [w396] -> w392
              tunnel: w394 -> [w395] mode=indexing
              n114 = Enqueue Element At Opposite End(queue=w398, element=w395, error in (no error)=w397) -> (error out=w396:errorcluster)  [unwired: 1 in, 2 out]
            }
          }
        }
        n115 = call "ElapsedTime2.vi"("error in (no error)"=w371, "Mode (Update)"=enum16{"Update", "Init"}."Init") -> ("error out"=w366:errorcluster)  [unwired: 8 in, 1 out]
      }
      frame "Get Block" {
        # "LT&RT won't be accurate unless PIXIE is stopped."
        # "Problem: PIXIE & FCs not synched."
        n116 = call-poly <vilib>:"DAQmx Read.vi"("task/channels in"=w461, "number of samples per channel"=-1, "timeout"=10.0, "error in"=w449) -> ("task out"=w443:refnum<k21>, "data"=w453:waveform(dbl)[], "error out"=w429:errorcluster)  [unwired: 9 out]
        n117 = call "ProcessFCCurrentsLE.vi"("FC Data"=w453, "Bouncer Settings"=w444, "FC Offset"="FC Offset") -> ("Mean Currents"=w451:dbl[], "Output Waveforms"=w452:waveform(dbl)[])  [unwired: 7 in]
        n118 = Index Array(array=w452) -> (element #1=→"HE 12C Cup":waveform(dbl), element #2=→"LE 12C Cup":waveform(dbl), element #3=w432:waveform(dbl), element #4=w431:waveform(dbl), element #5=→"LE 13C Cup":waveform(dbl), element #6=→"Bouncer V":waveform(dbl), element #7=→"Bouncer I":waveform(dbl))  [unwired: 7 in]
        "HE 13CL Cup" <- w431
        "HE 13CH Cup" <- w432
        n119 = call <vilib>:"DAQmx Stop Task.vi"("task/channels in"=w443, "error in"=w429) -> ("task out"=w442:refnum<k21>, "error out"=w441:errorcluster)  [unwired: 12 in]
        n120 = call <vilib>:"DAQmx Start Task.vi"("task/channels in"=w442, "error in"=w441) -> ("task out"=w424:refnum<k21>, "error out"=w428:errorcluster)  [unwired: 12 in]
        n121 = Index Array(array=w451) -> (element #1=w437:dbl, element #2=w439:dbl, element #3=w404:dbl, element #4=w400:dbl, element #5=w438:dbl)  [unwired: 5 in]
        n122 = call "PixieGetData.vi"("error IO"=w428) -> ("error out"=w427:errorcluster, "PixieTimes"=w422:T13, "Histogram Data"=w423:u32[][])  [unwired: 8 in]
        "Block Spectrum" <- w423
        n123 = property on="Block Spectrum" class="WFGraph (strict)"() -> ("CrsrList"=w458:T14)  [unwired: 2 in, 2 out]
        n124 = Add(1:w431, 2:w432) -> (0:→"HE 13 SUM":waveform(dbl))  [unwired: 1 in, 1 out]
        n125 = Divide(1:w431, 2:w432) -> (0:→"HE 13 Ratio":waveform(dbl))  [unwired: 1 in, 1 out]
        n126 = call "PixieCalcCountData.vi"("PixieTimes"=w422, "Histogram Data"=w423, "CrsrList"=w458) -> ("Count Data"=w457:T15)  [unwired: 8 in]
        n127 = Unbundle By Name(w457) -> ("Ch0 Counts"=→"Ch0 Counts":u32, "Ch1 Counts"=w412:u32, "Ch0 Rate"=→"Ch0 Rate":dbl, "Ch1 Rate"=→"Ch1 Rate":dbl, "Ch0 Cor Rate"=→"DT Corrected Rate Ch0":dbl, "Ch1 Cor Rate"=→"DT Corrected Rate Ch1":dbl, "Ch1 Cor LT"=w410:dbl)
        "Ch1 Counts" <- w412
        n128 = Unbundle By Name(w422) -> ("CH0 LT"=→"Ch0 LT":dbl, "CH1 LT"=→"Ch1 LT":dbl, "CH0 SFDT"=→"CH0 SFDT":dbl, "CH1 SFDT"=→"CH1 SFDT":dbl, "CH0 GDT"=→"CH0 GDT":dbl, "CH1 GDT"=→"CH1 GDT":dbl, "Run time [s]"=w411:dbl)
        "Run time [s]" <- w411
        n129 = call "LoopTime.vi"("error in (no error)"=w427) -> ("error out"=w405:errorcluster, "LoopTime"=→"LoopTime":u32)  [unwired: 9 in]
        n130 = call "InsertBlockData.vi"("C12LE"=w439, "C12"=w437, "Block Data In"=w436, "C13H"=w404, "C13L"=w400, "C13LE"=w438, "Counts"=w412, "LT"=w410, "RT"=w411) -> ("Block Data Out"=w459:T10)  [unwired: 6 in]
      }
      frame "Check Data" {
        # "Removing bad data won't work\nbecause counts, lt, rt are cumulative"
        # "Check block data"
        # "Check data quality\n    add to run data if good\n    discard, increment bad block counter\n     get new block if bad"
        n131 = call "ElapsedTime2.vi"("error in (no error)"=w476, "Mode (Update)"=enum16{"Update", "Init"}."Update") -> ("error out"=w468:errorcluster, "Elapsed Time"=→"GetBlocktime":u32)  [unwired: 8 in]
        n132 = case shown="True" "Stop DAQ" {
          tunnel: w486 -> [w496 w499]
          tunnel: [w496 w498] -> w464
          frame False {
          }
          frame True {
            n133 = Enqueue Element(queue=w499, element=PixieKeithleyDAQstates."Stop DAQ" ("Next State")) -> (queue out=w498:refnum<queue>)  [unwired: 1 in, 3 out]
          }
        }
        n134 = Unbundle By Name(w478) -> ("C12"=w490:dbl[])
        n135 = Unbundle By Name(w485) -> ("C12 Limit"=w491:dbl, "Max BadBlocks"=w487:u8)
        n136 = Delete From Array(array=w490) -> (deleted portion=w489:dbl)  [unwired: 2 in, 1 out]
        n137 = Greater?(x=w489, y=w491) -> (0:w488:bool)
        "Good Block" <- w488
        n138 = case shown="True" "Clear" {
          tunnel: w464 -> [w492 w495]
          tunnel: [w492 w494] -> w463
          frame False {
          }
          frame True {
            n139 = Enqueue Element(queue=w495, element=PixieKeithleyDAQstates."Clear" ("Next State")) -> (queue out=w494:refnum<queue>)  [unwired: 1 in, 3 out]
          }
        }
        n140 = case shown="True" w488 {
          tunnel: [w511 w521] -> w479
          tunnel: w480 -> [w512 w522]
          tunnel: w478 -> [w501 w520]
          tunnel: w487 -> [w510 _]
          tunnel: w463 -> [w508 w524]
          tunnel: [w500 w520] -> w477
          frame False {
            w505 = T9[] [enum."Wait", enum."Get Block", enum."Check Data"] items=["Idle", "Initialize", "Bouncer", "Load Wheel", "Load Sample", "Start Run", "Clear", "Wait", "Get Block", "Check Data", "Check Run", "Check Sample", "Analyse and Display", "Stop DAQ", "Stop FC", "Log Data", "Stop"]
            w507 = T9[] [enum."Stop DAQ"] items=["Idle", "Initialize", "Bouncer", "Load Wheel", "Load Sample", "Start Run", "Clear", "Wait", "Get Block", "Check Data", "Check Run", "Check Sample", "Analyse and Display", "Stop DAQ", "Stop FC", "Log Data", "Stop"]
            # "Stopping for too many badblocks won't work"
            # "Bad Block"
            n141 = Unbundle By Name(w512) -> ("BadBlocks"=w504:u8)
            n142 = Decrement(x=w510) -> (x-1=w503:u8)
            n143 = Increment(x=w504) -> (x+1=w502:u8)
            n144 = disable-structure shown="Enabled" {
              disable-tunnel: w501 -> [w514 w515]
              disable-tunnel: [w513 w515] -> w500
              frame Disabled {
                # "Remove bad data"
                n145 = call "DeleteBlockData.vi"("Block Data In"=w514) -> ("Block Data Out"=w513:T10)  [unwired: 10 in]
              }
              frame Enabled {
              }
            }
            n146 = Bundle By Name(cluster=w512, "BadBlocks"=w502) -> (w511:T7)
            n147 = Greater Or Equal?(x=w502, y=w503) -> (x >= y?=w509:bool)
            n148 = Select(t=w507, s=w509, f=w505) -> (s? t:f=w506:T9[])
            n149 = for {
              tunnel: w506 -> [w517] mode=indexing
              tunnel: w508 -> [w516]
              n150 = Enqueue Element(queue=w516, element=w517) -> ()  [unwired: 1 in, 4 out]
            }
          }
          frame True {
            # "Good block"
            n151 = call "PKDAQAppendBlockDataCont.vi"("Run Summary"=w522, "Block Data"=w520) -> ("Transmission"=w519:dbl, "Run Summary Out"=w521:T7)  [unwired: 8 out]
            n152 = Enqueue Element(queue=w524, element=PixieKeithleyDAQstates."Check Run") -> ()  [unwired: 1 in, 4 out]
            n153 = Negate(x=w519) -> (-x=→"Transmission":dbl)
          }
        }
        "Summary Data" <- w479
      }
      frame "Check Run" {
        # "Done with run?"
        n154 = Unbundle By Name(w526) -> ("Max Counts"=w559:u32, "WarmupTime"=w529:dbl, "Warmup"=w531:bool, "Max Runtime (s)"=w530:dbl, "Tuning"=w532:bool)
        n155 = Unbundle By Name(w556) -> ("Counts"=w557:u32, "LT"=w528:dbl)
        n156 = Select(t=w529, s=w531, f=w530) -> (s? t:f=w533:dbl)
        n157 = Not(x=w532) -> (.not. x?=w543:bool)
        n158 = Greater Or Equal?(x=w557, y=w559) -> (x >= y?=w555:bool)
        n159 = Greater Or Equal?(x=w528, y=w533) -> (x >= y?=w554:bool)
        n160 = Or(x=w555, y=w554) -> (x .or. y?=w544:bool)
        n161 = And(x=w544, y=w543) -> (x .and. y?=w542:bool)
        n162 = case shown="True" w542 {
          tunnel: [w564 w570] -> w553
          tunnel: w547 -> [_ w569]
          tunnel: w549 -> [w563 w568]
          tunnel: [w563 w567] -> w540
          tunnel: w531 -> [w562 w566]
          tunnel: [w562 w565] -> w527
          frame False {
            w564 = T9[] [enum."Analyse and Display", enum."Wait", enum."Get Block", enum."Check Data"] items=["Idle", "Initialize", "Bouncer", "Load Wheel", "Load Sample", "Start Run", "Clear", "Wait", "Get Block", "Check Data", "Check Run", "Check Sample", "Analyse and Display", "Stop DAQ", "Stop FC", "Log Data", "Stop"]
          }
          frame True {
            n163 = case shown="True" w566 {
              selector: w566 -> [w571 _]
              tunnel: [w579 w582] -> w570
              tunnel: w569 -> [w577 _]
              tunnel: w568 -> [w576 w581]
              tunnel: [w575 w581] -> w567
              tunnel: [w571 w580] -> w565
              frame False {
                w579 = T9[] [enum."Analyse and Display", enum."Stop DAQ"] items=["Idle", "Initialize", "Bouncer", "Load Wheel", "Load Sample", "Start Run", "Clear", "Wait", "Get Block", "Check Data", "Check Run", "Check Sample", "Analyse and Display", "Stop DAQ", "Stop FC", "Log Data", "Stop"]
                # "Increment \"runs completed"
                n164 = Index Array(array=w576, index (row)=w577, index (col)=0 ("disabled index (col)")) -> (element=w578:i32)
                n165 = Increment(x=w578) -> (x+1=w572:i32)
                n166 = Replace Array Subset(array=w576, new element=w572, index (row)=w577, index (col)=0 ("disabled index (col)")) -> (w575:i32[][])
              }
              frame True {
                w580 = FALSE
                w582 = T9[] [enum."Analyse and Display", enum."Clear"] items=["Idle", "Initialize", "Bouncer", "Load Wheel", "Load Sample", "Start Run", "Clear", "Wait", "Get Block", "Check Data", "Check Run", "Check Sample", "Analyse and Display", "Stop DAQ", "Stop FC", "Log Data", "Stop"]
                n167 = local write "Warmup"(w580) -> ()
              }
            }
          }
        }
        n168 = for {
          tunnel: w534 -> [w561]
          tunnel: w553 -> [w560] mode=indexing
          n169 = Enqueue Element(queue=w561, element=w560) -> ()  [unwired: 1 in, 4 out]
        }
        n170 = Index Array(array=w540, index (col)=0 ("disabled index (col)")) -> (element=→"Meas":i32[])  [unwired: 1 in]
        n171 = Bundle By Name(cluster=w526, "Warmup"=w527) -> (w525:T1)
      }
      frame "Analyse and Display" {
        # "Increment\nBad Block\nCounter"
        n172 = disable-structure shown="Disabled" {
          frame Disabled {
            n173 = Select(t=u8 2, s="Autoscale", f=u8 0) -> (s? t:f=w647:u8)
            n174 = property on="Ratios" class="WFChart (strict)"("YScale.ScaleFit"=w647) -> ()  [unwired: 2 in, 2 out]
            n175 = property on="Currents & Counts" class="WFChart (strict)"("YScale.ScaleFit"=w647) -> ()  [unwired: 2 in, 2 out]
            n176 = property on="LE Currents" class="WFChart (strict)"("YScale.ScaleFit"=w647) -> ()  [unwired: 2 in, 2 out]
          }
          frame Enabled {
          }
        }
        n177 = case shown="True" "Clear Charts" {
          frame False {
          }
          frame True {
            n178 = property on="Currents & Counts" class="WFChart (strict)"("History Data"=cluster{"C14Rate":dbl, "C12":dbl, dbl}[] []) -> ()  [unwired: 2 in, 2 out]
            n179 = property on="Ratios" class="WFChart (strict)"("History Data"=T11 []) -> ()  [unwired: 2 in, 2 out]
            n180 = property on="LE Currents" class="WFChart (strict)"("History Data"=cluster{"C13LE":dbl, "C12LE":dbl}[] []) -> ()  [unwired: 2 in, 2 out]
          }
        }
        n181 = call "PKDAQRunningAvg.vi"("Block Data"=w608, "CountPoints"="CountPoints", "CurPoints"="CurPoints") -> ("RunningAverages"=w585:T7)  [unwired: 8 out]
        "RunningAverages" <- w585
        n182 = call "CalcRatiosBouncer.vi"("Run Summary"=w633) -> ("Run Ratios"=w635:T8)  [unwired: 10 out]
        "Run Average Ratios" <- w635
        n183 = call "CalcRatiosBouncer.vi"("Run Summary"=w585) -> ("Run Ratios"=w642:T8)  [unwired: 10 out]
        "Moving Average Ratios" <- w642
        n184 = Unbundle By Name(w635) -> ("DTfrac"=→"Dead time fraction":dbl, "C14/12"=w641:dbl, "d13C"=w638:dbl)
        n185 = Unbundle By Name(w642) -> ("C14/12"=w640:dbl, "d13C"=w637:dbl, "C14Rate"=w605:dbl, "C13H/L"=→"13C H/L":dbl)
        n186 = Unbundle By Name(w585) -> ("C13H"=w593:dbl, "C13L"=w591:dbl, "C12"=w595:dbl, "C13LE"=w592:dbl, "C12LE"=w594:dbl)
        "C12" <- w595
        "C12LE" <- w594
        "C13H" <- w593
        "C13LE" <- w592
        "C13L" <- w591
        n187 = Add(x=w593, y=w591) -> (x+y=w597:dbl)
        "C13" <- w597
        n188 = Bundle("C14/12"=w641, "C14/12"=w640, "d13C"=w638, "d13C"=w637) -> (→"Ratios":T2)  [unwired: 1 out]
        n189 = Less?(x=w595, y=1e-06) -> (x < y?=w601:bool)
        n190 = Multiply(x=w595, y=1000000.0) -> (x*y=w604:dbl)
        n191 = Multiply(x=w597, y=100000000.0) -> (x*y=w615:dbl)
        n192 = Multiply(x=w597, y="C13 2") -> (x*y=w609:dbl)
        n193 = Multiply(x=w595, y="C12 2") -> (x*y=w622:dbl)
        n194 = Multiply(x="C13LE 2", y=w592) -> (x*y=w624:dbl)
        n195 = Multiply(x=w594, y="C12LE 2") -> (x*y=w623:dbl)
        n196 = Bundle(w604, w615) -> (→"Currents (uA)":cluster{dbl, dbl})  [unwired: 1 out]
        n197 = Bundle("C14Rate"=w605, w609, w622) -> (→"Currents & Counts":cluster{"C14Rate":dbl, dbl, dbl})  [unwired: 1 out]
        n198 = Bundle(w624, w623) -> (→"LE Currents":cluster{dbl, dbl})  [unwired: 1 out]
        n199 = call "C13HLAverager.vi"("Block Data"=w608, "low limit"="low limit", "CurPoints"="C13HLPoints") -> ("13CCurrent"=w617:bool, "C13HL"=w619:dbl)  [unwired: 7 in]
        "Split Cup Good" <- w617
        n200 = shared-variable "My Computer\\NOSAMSPixieDAQVars.lvlib\\C13HL"(w619, error in=w588) -> (error out=w586:errorcluster)
        n201 = shared-variable "My Computer\\NOSAMSPixieDAQVars.lvlib\\C13HLGood"(w617, error in=w586) -> (error out=w584:errorcluster)
        n202 = shared-variable "My Computer\\NOSAMSPixieDAQVars.lvlib\\CountRate"(w605, error in=w584) -> (error out=w583:errorcluster)
        n203 = shared-variable "My Computer\\NOSAMSPixieDAQVars.lvlib\\C12Cur"(w595, error in=w583) -> (error out=w590:errorcluster)
        n204 = shared-variable "My Computer\\NOSAMSPixieDAQVars.lvlib\\C13"(w597, error in=w590) -> (error out=w589:errorcluster)
        n205 = shared-variable "My Computer\\NOSAMSPixieDAQVars.lvlib\\C12LE"(w594, error in=w589) -> (error out=w587:errorcluster)
        n206 = case shown="True" w601 {
          tunnel: w600 -> [_ w654]
          tunnel: [0 w653] -> w598
          frame False {
          }
          frame True {
            n207 = Increment(x=w654) -> (x+1=w653:i32)
          }
        }
      }
      frame "Check Sample" {
        # "End of Run"
        # "Low current counter"
        n208 = Flush Queue(queue=w673) -> (queue out=w668:refnum<queue>)  [unwired: 1 in, 2 out]
        n209 = Greater?(x=w663, y=3800) -> (0:w665:bool)
        n210 = call "FindNextTarget.vi"("error in (no error)"=w659, "CurPos"=w657, "Runlist"=w655, "RunsDone"=w656) -> ("error out"=w658:errorcluster, "NextPos"=w660:i32)  [unwired: 6 in]
        n211 = case shown="-1, Default" w660 {
          selector: w660 -> [_ w707]
          tunnel: [PixieKeithleyDAQstates."Idle" ("element") PixieKeithleyDAQstates."Load Sample" ("States")] -> w674
          tunnel: [w689 w707] -> w667
          tunnel: w665 -> [w688 _]
          tunnel: [0 w706] -> w664
          tunnel: w663 -> [_ w706]
          tunnel: w658 -> [w686 w705]
          tunnel: [w680 w705] -> w662
          frame -1, Default {
            w689 = 0 ("index of element")
            # "No current shutdown"
            n212 = case shown="True" w688 {
              tunnel: w686 -> [w698 w703]
              tunnel: [w697 w702] -> w685
              frame False {
                n213 = property on="wheelname" class="Str"() -> ("Value"=w696:string)  [unwired: 2 in, 2 out]
                n214 = Concatenate Strings(w696, " just finished. Woo hoo!") -> (w699:string)
                n215 = call "SendtoSlack.vi"("error in (no error)"=w698, "buffer"=w699) -> ("error out"=w697:errorcluster)  [unwired: 7 in, 2 out]
              }
              frame True {
                n216 = property on="wheelname" class="Str"() -> ("Value"=w700:string)  [unwired: 2 in, 2 out]
                n217 = Concatenate Strings(w700, " Doh! Shut down due to no current!" ("string")) -> (w701:string)
                n218 = call "SendtoSlack.vi"("error in (no error)"=w703, "buffer"=w701) -> ("error out"=w702:errorcluster)  [unwired: 7 in, 2 out]
              }
            }
            n219 = case shown="True" "Source Auto-shutdown" {
              tunnel: w685 -> [w691 w693]
              tunnel: [w691 w692] -> w681
              frame False {
              }
              frame True {
                n220 = shared-variable "My Computer\\NOSAMSPixieDAQVars.lvlib\\ResEnable"(FALSE ("ResEnable"), error in=w693) -> (error out=w692:errorcluster)
              }
            }
            n221 = shared-variable "My Computer\\NOSAMSPixieDAQVars.lvlib\\PosReq"(w689, error in=w681) -> (error out=w683:errorcluster)
            n222 = shared-variable "My Computer\\NOSAMSPixieDAQVars.lvlib\\Auto"(FALSE ("Auto"), error in=w683) -> (error out=w680:errorcluster)
          }
          frame 0..133 {
          }
        }
        n223 = Enqueue Element(queue=w668, element=w674) -> ()  [unwired: 2 in, 3 out]
      }
      frame "Log Data" {
        n224 = call "ElapsedTime.vi"("error in (no error)"=w740) -> ("error out"=w739:errorcluster, "Elapsed Time"=w738:dbl)  [unwired: 1 in, 8 out]
        "Elapsed time" <- w738
        n225 = call-poly <vilib>:"DAQmx Read.vi"("task/channels in"=w745, "error in"=w739) -> ("task out"=w744:refnum<k21>, "data"=w737:u32, "error out"=w743:errorcluster)  [unwired: 1 in, 10 out]
        "SCA Counts" <- w737
        n226 = Divide(x=w737, y=w738) -> (x/y=→"SCA Rate":dbl)
        n227 = call <vilib>:"DAQmx Stop Task.vi"("task/channels in"=w744, "error in"=w743) -> ("task out"=w742:refnum<k21>, "error out"=w741:errorcluster)  [unwired: 12 out]
        n228 = call <vilib>:"DAQmx Stop Task.vi"("task/channels in"=w748, "error in"=w741) -> ("task out"=w747:refnum<k21>, "error out"=w717:errorcluster)  [unwired: 12 out]
        n229 = shared-variable "My Computer\\NOSAMSPixieDAQVars.lvlib\\C13HLGood"(FALSE ("C13HLGood"), error in=w717) -> (error out=w716:errorcluster)
        n230 = Index Array(array=w727, index (row) #1=w710, index (col) #1=1 ("disabled index (col)"), index (row) #2=w710, index (col) #2=3 ("disabled index (col)")) -> (element #1=w729:string, element #2=w728:string)
        n231 = Index Array(array=w712, index (row)=w710, index (col)=0 ("disabled index (col)")) -> (element=w711:i32)
        n232 = Bundle("index of element"=w710, "element"=w711, "format string"=w729, "format string"=w728) -> (w709:T16)  [unwired: 1 in]
        n233 = property on="Results path" class="Path"() -> ("Value"=w720:path)  [unwired: 2 in, 2 out]
        n234 = property on="wheelname" class="Str"() -> ("Value"=w719:string)  [unwired: 2 in, 2 out]
        n235 = call "LogFudgerData.vi"("Run Ratios"=w723, "error in (no error)"=w716, "Run Summary"=w724, "Sample Data"=w709, "Log File Path"=w720) -> ("error out"=w721:errorcluster)  [unwired: 5 in, 1 out]
        n236 = call "CopyResultsFile.vi"("error in (no error)"=w721, "Wheelname"=w719, "Server Path"="Server Results Directory", "source path"=w720) -> ("error out"=w715:errorcluster)  [unwired: 7 in]
        n237 = disable-structure shown="Disabled" {
          disable-tunnel: w715 -> [w750 w759]
          disable-tunnel: [w749 w759] -> w714
          frame Disabled {
            n238 = case shown="Error" w750 {
              selector: w750 -> [w751 w753]
              tunnel: [w751 w756] -> w749
              frame No Error {
              }
              frame Error {
                w752 = T12 0 items=["no dialog", "OK message", "continue or stop message", "OK message + warnings", "continue/stop + warnings"] ("type of dialog (OK msg:1)")
                n239 = call <vilib>:"General Error Handler.vi"("type of dialog (OK msg:1)"=w752, "error in (no error)"=w753) -> ("message"=w757:string, "error out"=w755:errorcluster)  [unwired: 9 in, 3 out]
                n240 = call <vilib>:"Clear Errors.vi"("error in (no error)"=w755) -> ("error out"=w754:errorcluster)  [unwired: 6 in]
                n241 = Write to Text File(file (use dialog)=path "", text=w757, error in=w754) -> (error out=w756:errorcluster)  [unwired: 1 in, 2 out]
              }
            }
          }
          frame Enabled {
          }
        }
      }
      frame "Stop DAQ" {
        n242 = call "PixieStopACQ.vi"("error in (no error)"=w774) -> ("error out"=w778:errorcluster)  [unwired: 10 out]
        n243 = call "PixieCheckRunStatus.vi"("error in (no error)"=w778) -> ("error out"=w761:errorcluster, "run finished"=w777:bool)  [unwired: 1 in, 8 out]
        n244 = case shown="True" w777 {
          tunnel: w776 -> [w782 w786]
          tunnel: w763 -> [_ w784]
          frame False {
            n245 = Enqueue Element(queue=w782, element=PixieKeithleyDAQstates."Stop DAQ" ("Next State")) -> ()  [unwired: 1 in, 4 out]
          }
          frame True {
            n246 = Unbundle By Name(w784) -> ("Tuning"=w783:bool)
            n247 = case shown="False" w783 {
              tunnel: [w787 w788] -> w785
              frame False {
                w787 = T9[] [enum."Wait", enum."Get Block", enum."Check Data", enum."Analyse and Display", enum."Wait", enum."Stop FC", enum."Log Data", enum."Check Sample"] items=["Idle", "Initialize", "Bouncer", "Load Wheel", "Load Sample", "Start Run", "Clear", "Wait", "Get Block", "Check Data", "Check Run", "Check Sample", "Analyse and Display", "Stop DAQ", "Stop FC", "Log Data", "Stop"]
              }
              frame True {
                w788 = T9[] [enum."Wait", enum."Get Block", enum."Check Data", enum."Analyse and Display", enum."Wait", enum."Stop FC", enum."Idle"] items=["Idle", "Initialize", "Bouncer", "Load Wheel", "Load Sample", "Start Run", "Clear", "Wait", "Get Block", "Check Data", "Check Run", "Check Sample", "Analyse and Display", "Stop DAQ", "Stop FC", "Log Data", "Stop"]
              }
            }
            n248 = for {
              tunnel: w786 -> [w790]
              tunnel: w785 -> [w789] mode=indexing
              n249 = Enqueue Element(queue=w790, element=w789) -> ()  [unwired: 1 in, 4 out]
            }
          }
        }
        n250 = shared-variable "My Computer\\NOSAMSPixieDAQVars.lvlib\\C13HLGood"(FALSE ("C13HLGood"), error in=w761) -> (error out=w760:errorcluster)
      }
      frame "Clear" {
        n251 = call "PixieStopACQ.vi"("error in (no error)"=w805) -> ("error out"=w809:errorcluster)  [unwired: 10 out]
        n252 = call "PixieCheckRunStatus.vi"("error in (no error)"=w809) -> ("error out"=w792:errorcluster, "run finished"=w808:bool)  [unwired: 1 in, 8 out]
        n253 = case shown="True" w808 {
          tunnel: w807 -> [w813 w815]
          frame False {
            n254 = Enqueue Element(queue=w813, element=PixieKeithleyDAQstates."Clear" ("Next State")) -> ()  [unwired: 1 in, 4 out]
          }
          frame True {
            w814 = T9[] [enum."Stop FC", enum."Start Run"] items=["Idle", "Initialize", "Bouncer", "Load Wheel", "Load Sample", "Start Run", "Clear", "Wait", "Get Block", "Check Data", "Check Run", "Check Sample", "Analyse and Display", "Stop DAQ", "Stop FC", "Log Data", "Stop"]
            n255 = for {
              tunnel: w815 -> [w817]
              tunnel: w814 -> [w816] mode=indexing
              n256 = Enqueue Element(queue=w817, element=w816) -> ()  [unwired: 1 in, 4 out]
            }
          }
        }
        n257 = shared-variable "My Computer\\NOSAMSPixieDAQVars.lvlib\\C13HLGood"(FALSE ("C13HLGood"), error in=w792) -> (error out=w791:errorcluster)
      }
      frame "Stop FC" {
        n258 = shared-variable "My Computer\\NOSAMSPixieDAQVars.lvlib\\C13HLGood"(FALSE ("C13HLGood"), error in=w819) -> (error out=w818:errorcluster)
        n259 = call <vilib>:"DAQmx Stop Task.vi"("task/channels in"=w829, "error in"=w818) -> ("task out"=w828:refnum<k21>, "error out"=w823:errorcluster)  [unwired: 12 out]
        n260 = call <vilib>:"DAQmx Stop Task.vi"("task/channels in"=w825, "error in"=w823) -> ("task out"=w824:refnum<k21>, "error out"=w822:errorcluster)  [unwired: 12 out]
      }
      frame "Stop" {
        n261 = Enqueue Element(queue=w852, element=PixieKeithleyDAQstates."Stop" ("Next State")) -> ()  [unwired: 1 in, 4 out]
      }
    }
    n262 = Equal?(x=w67, y=PixieKeithleyDAQstates."Stop" ("States")) -> (x = y?=w80:bool)
  }
  n263 = call <vilib>:"DAQmx Stop Task.vi"("task/channels in"=w14, "error in"=w12) -> ("task out"=w13:refnum<k21>, "error out"=w11:errorcluster)  [unwired: 12 out]
  n264 = call <vilib>:"DAQmx Clear Task.vi"("task in"=w13, "error in"=w11) -> ("error out"=w10:errorcluster)  [unwired: 13 in]
  n265 = call <vilib>:"DAQmx Stop Task.vi"("task/channels in"=w9, "error in"=w10) -> ("task out"=w8:refnum<k21>, "error out"=w7:errorcluster)  [unwired: 12 out]
  n266 = call <vilib>:"DAQmx Clear Task.vi"("task in"=w8, "error in"=w7) -> ("error out"=w15:errorcluster)  [unwired: 13 in]
  n267 = call <vilib>:"DAQmx Clear Task.vi"("task in"=w36, "error in"=w15) -> ("error out"=w23:errorcluster)  [unwired: 13 out]
  n268 = call <vilib>:"DAQmx Clear Task.vi"("task in"=w21, "error in"=w23) -> ("error out"=w22:errorcluster)  [unwired: 13 out]
  n269 = Release Queue(queue=w31, error in (no error)=w22) -> (error out=w27:errorcluster)  [unwired: 3 out]
  n270 = call <vilib>:"General Error Handler.vi"("error in (no error)"=w27) -> ()  [unwired: 1 in, 14 out]
